vi "Do_Every_minute.vi"(1 "Ch Names":string[](array[string]), 2 "Values":dbl[](array[numeric]) format="%.2f") -> (0 "Scan Comments":string)   [LabVIEW 2017]
uses:
  Anemometry/Anemometry Sub Vis/Controls/In_Range.ctl
  ADAM Client/Sub VIs/ADAM Controls/Update_scan_value.ctl
  ADAM Client/Sub VIs/ADAM Controls/Traverse_Level_State.ctl
  ADAM Client/Sub VIs/ADAM Controls/Valco_valve_ph.ctl
  <vilib>/Analysis/baseanly.llb/Mean (DBL).vi
  Anemometry/Anemometry Sub Vis/Globals/EnFlo_Tunnel_Global.vi
  ADAM_Global.vi
  <vilib>/Analysis/NI_AALBase.lvlib
panel:
  in  "Kp":dbl=50.0 format="%#_13g"
  in  "Deadband Delta T":dbl=0.002 format="%#_13g"
  out "Max Delta T":dbl(graph)
  in  "Manual Control of Lamps":bool
  out "Power":dbl[][](graph)=[[0.00729, 0.18153463174730816, 0.17352738437348433, 1.6752433719500537, 8.231465735195274, 17.570357598383207, 23.099772817121426, 25.58386930448374, 25.31727725753219, 24.28926231541072, 18.717383219374323, 10.355253339797807, 2.7760273383248344, 0.3109897541921306, 0.08276881403435009, 0.06197], [0.04411, 0.1361526368018142, 0.04039202183336771, 1.5611636795339547, 8.176972694107874, 17.32000974741714, 24.257541358764026, 25.949153465972987, 26.01802540761648, 25.060373307424115, 18.284750328365213, 8.689831176707928, 2.642937641487066, 0.43219350072447926, -0.019957690739617468, 0.07351], [0.05478, 0.03446320268089581, 0.2086595806581808, 1.6919212249796047, 6.580368005180591, 14.333585185483123, 21.06810094963999, 23.709254571137723, 24.04768940379576, 21.01660820522005, 13.60443428327954, 6.2766496258038735, 1.7988963349022484, 0.2952877651784204, 0.05436788410934033, 0.1022], [0.04013, 0.06419557464541133, 0.2035068586120256, 1.3118741659450193, 4.7061387064566835, 9.009825946069038, 12.927700276268434, 17.003135081884164, 16.83885730812343, 12.902263313363814, 8.246161922417906, 4.035269404379355, 1.329605659745338, 0.24574055091433544, 0.012829784119986217, 0.08755], [0.04404, 0.022691144295571734, 0.19102098261858932, 0.8525411026079828, 2.2353542219792946, 3.966676465246214, 6.305347763088489, 8.17672908183636, 7.7348668140659, 5.703994479070454, 3.8329088824353237, 1.9256956625267279, 0.6611488869641811, 0.20508248283573002, 0.10119553469307395, 0.08441]]
  out "Temperature":dbl[][](graph)=[[0.00729, 0.18153463174730816, 0.17352738437348433, 1.6752433719500537, 8.231465735195274, 17.570357598383207, 23.099772817121426, 25.58386930448374, 25.31727725753219, 24.28926231541072, 18.717383219374323, 10.355253339797807, 2.7760273383248344, 0.3109897541921306, 0.08276881403435009, 0.06197], [0.04411, 0.1361526368018142, 0.04039202183336771, 1.5611636795339547, 8.176972694107874, 17.32000974741714, 24.257541358764026, 25.949153465972987, 26.01802540761648, 25.060373307424115, 18.284750328365213, 8.689831176707928, 2.642937641487066, 0.43219350072447926, -0.019957690739617468, 0.07351], [0.05478, 0.03446320268089581, 0.2086595806581808, 1.6919212249796047, 6.580368005180591, 14.333585185483123, 21.06810094963999, 23.709254571137723, 24.04768940379576, 21.01660820522005, 13.60443428327954, 6.2766496258038735, 1.7988963349022484, 0.2952877651784204, 0.05436788410934033, 0.1022], [0.04013, 0.06419557464541133, 0.2035068586120256, 1.3118741659450193, 4.7061387064566835, 9.009825946069038, 12.927700276268434, 17.003135081884164, 16.83885730812343, 12.902263313363814, 8.246161922417906, 4.035269404379355, 1.329605659745338, 0.24574055091433544, 0.012829784119986217, 0.08755], [0.04404, 0.022691144295571734, 0.19102098261858932, 0.8525411026079828, 2.2353542219792946, 3.966676465246214, 6.305347763088489, 8.17672908183636, 7.7348668140659, 5.703994479070454, 3.8329088824353237, 1.9256956625267279, 0.6611488869641811, 0.20508248283573002, 0.10119553469307395, 0.08441]]
  in  "Kp Lamps":dbl=50.0 format="%#_13g"
  in  "Averaging time in Seconds":dbl=200.0 format="%#_13g"
  in  "Disable Sending email to estates regarding Chilled water Temp":bool=TRUE
  in  "Max K Factor":dbl=16.0
  # "Control Parameters"
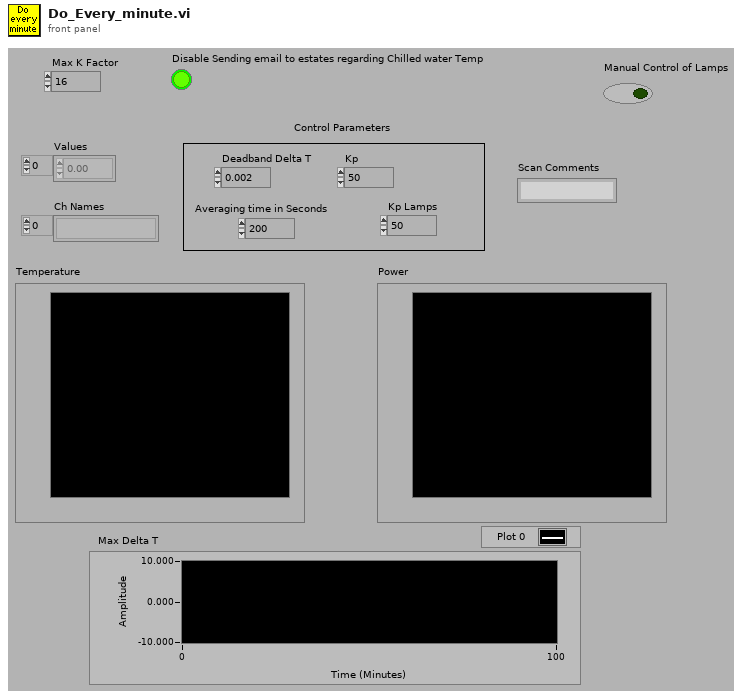
[diagram p1: front panel]
types:
  T1 = typedef "In_Range.ctl" = enum16{"%", "±", "% & ±"}
  T2 = typedef "Update_scan_value.ctl" = cluster{"Channel Name":string, "New Value":dbl}
  T3 = enum16{"Append to Global", "Read Global then Clear"}
  T4 = typedef "Traverse_Level_State.ctl" = enum16{"Running", "Complete"}
  T5 = cluster{"Bus Bar":string, "Connected Items":string[]}
  T6 = cluster{"Ch Name":string, "subarray":string[], "subarray":dbl[], i32, i32}
  T7 = typedef "Client_State_Cluster.ctl" = cluster{"Client Name":string, "Traverse level State":T4, "People to Email":string[], "Next Contact Time":dbl}
  T8 = typedef "Valco_valve_ph.ctl" = u16
  T9 = cluster{"second":i32, "minute":i32, "hour":i32, "day of month":i32, "month":i32, "year":i32, "day of week":i32, "day of year":i32, "is DST":i32}
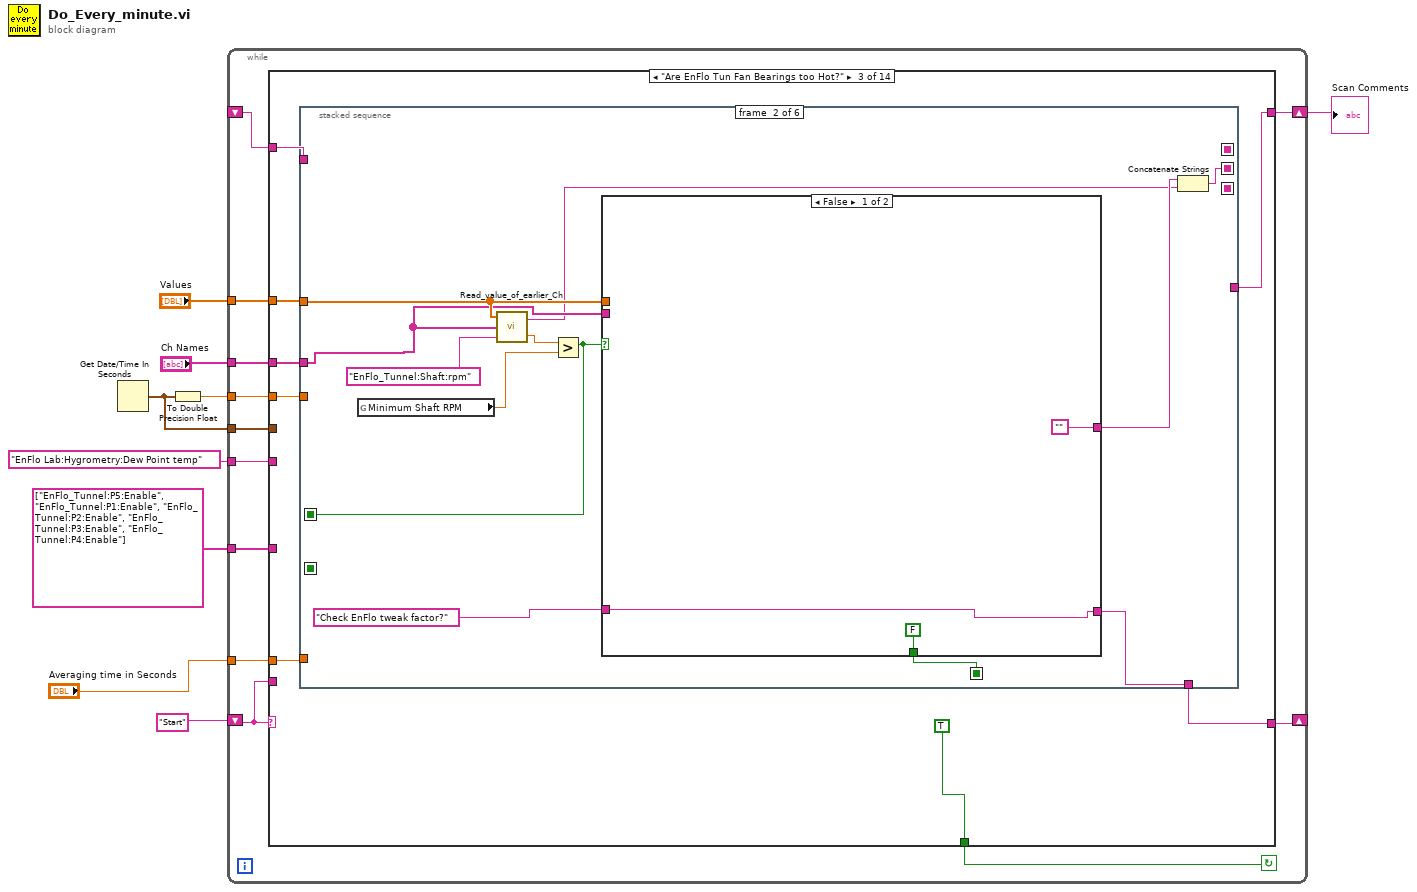
[diagram p0: block diagram]
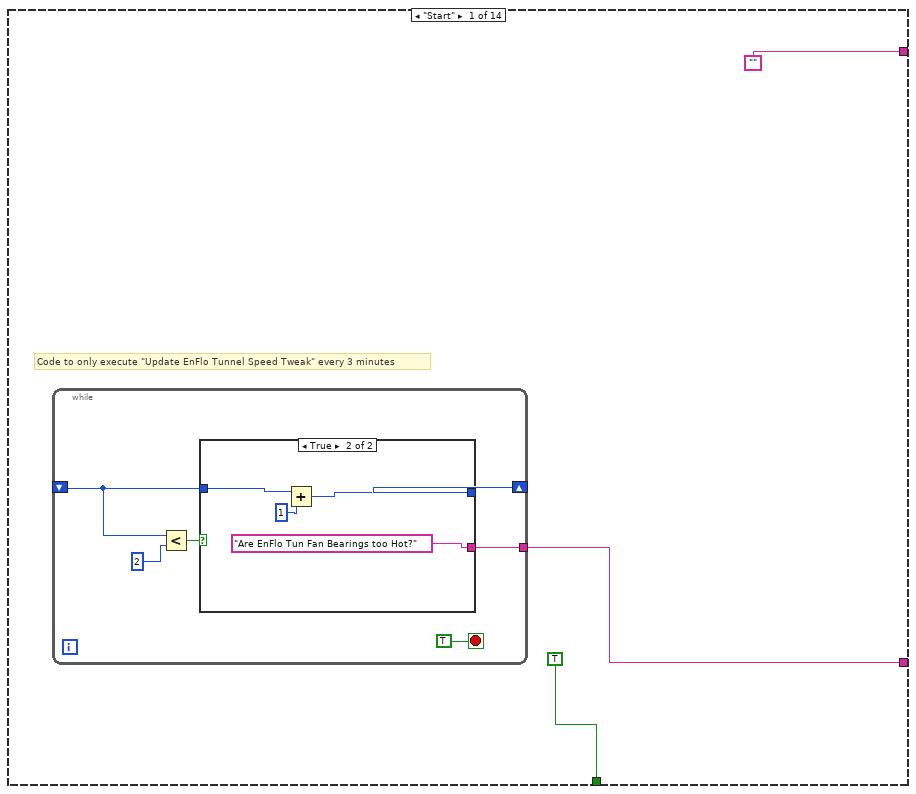
[diagram p2: hidden frame]
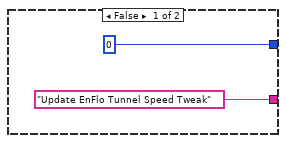
[diagram p3: hidden frame]
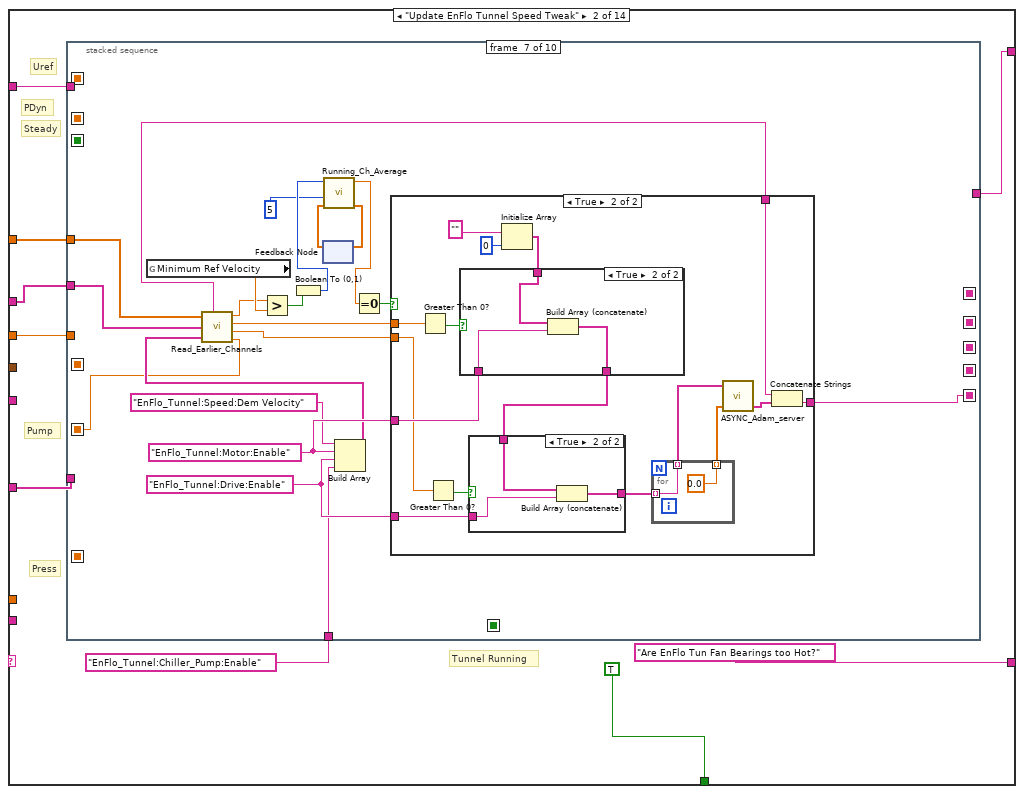
[diagram p4: hidden frame]
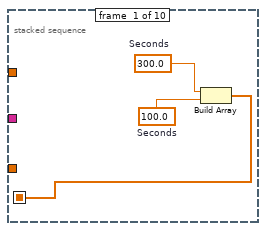
[diagram p5: hidden frame]
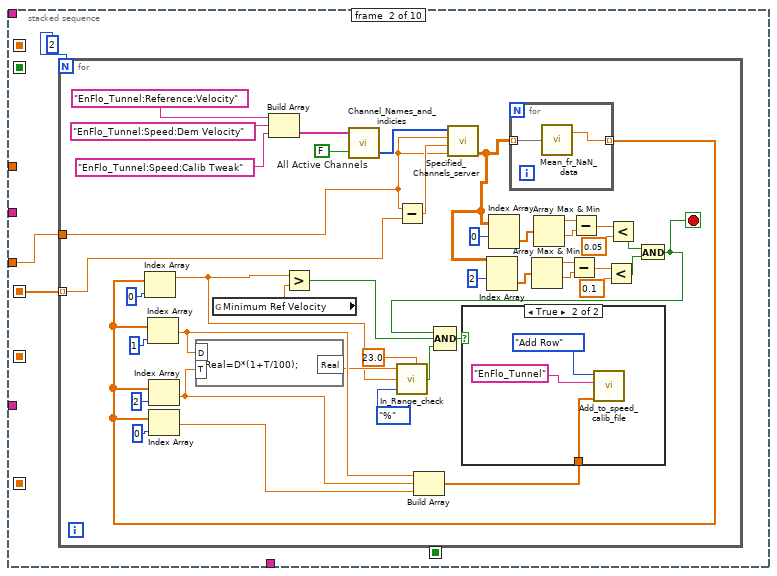
[diagram p6: hidden frame]
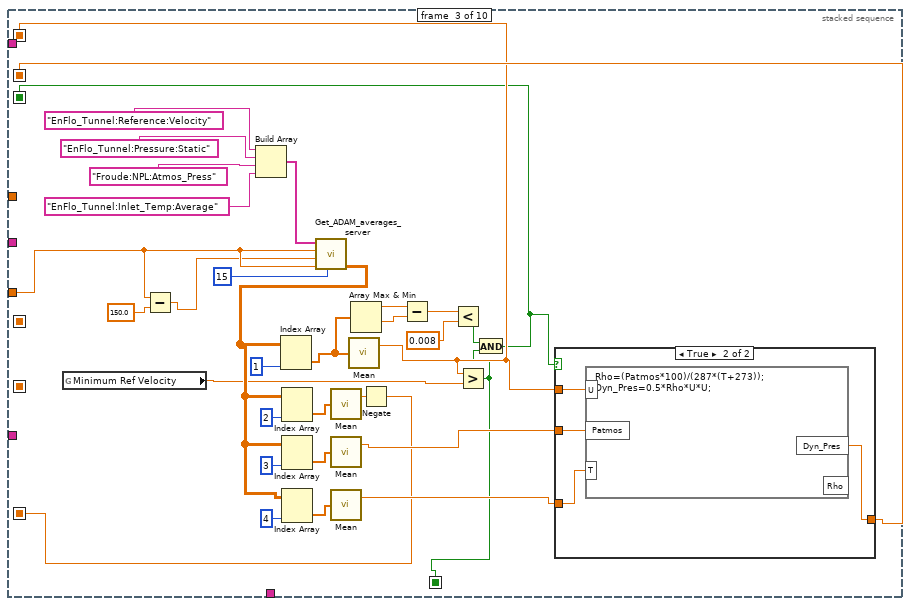
[diagram p8: hidden frame]
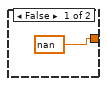
[diagram p9: hidden frame]
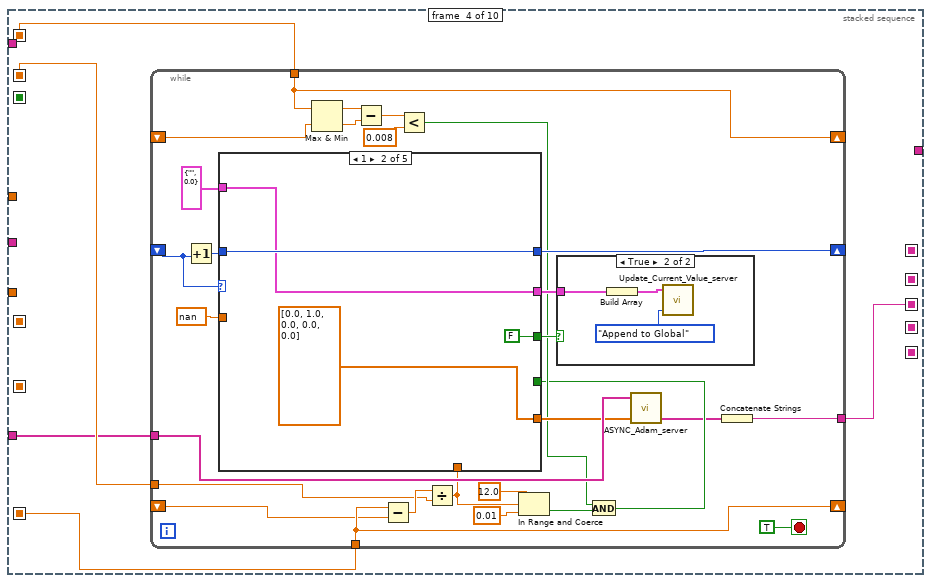
[diagram p10: hidden frame]
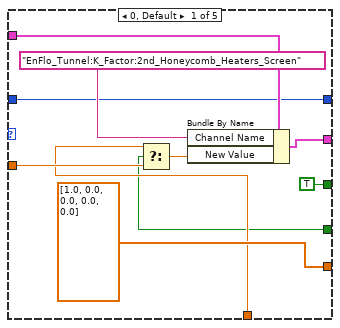
[diagram p12: hidden frame]
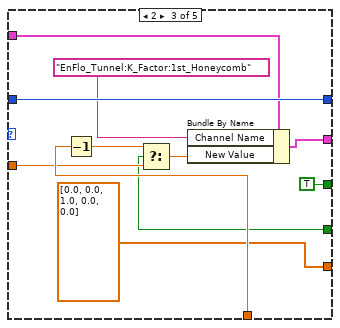
[diagram p13: hidden frame]
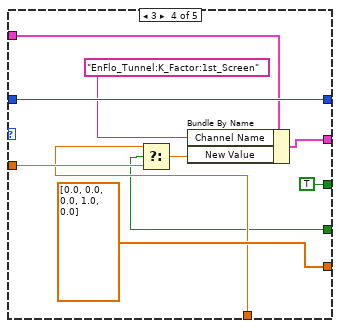
[diagram p14: hidden frame]
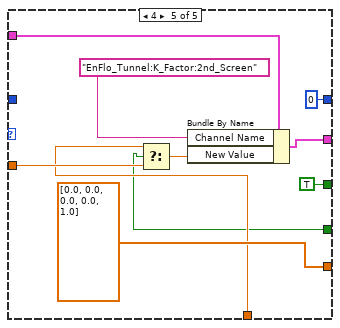
[diagram p15: hidden frame]
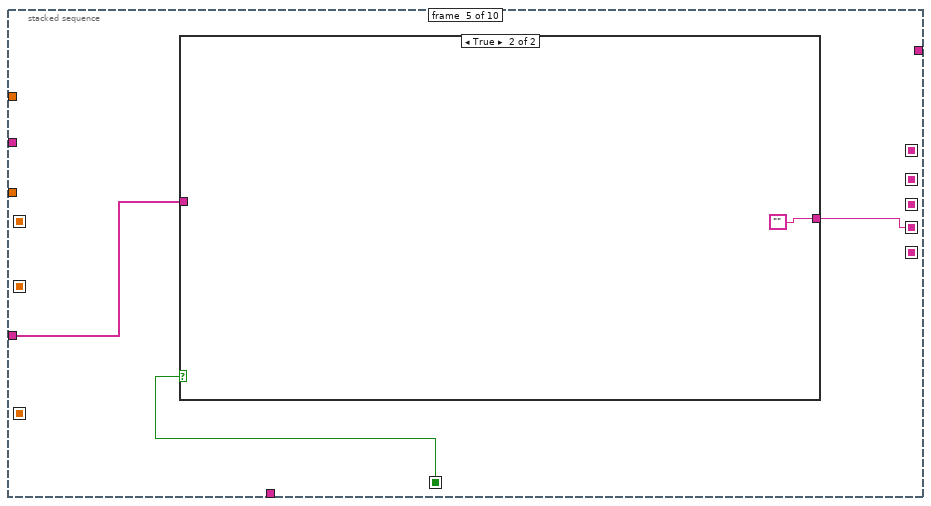
[diagram p16: hidden frame]
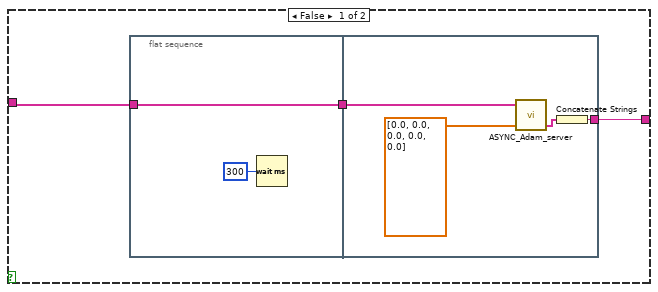
[diagram p17: hidden frame]
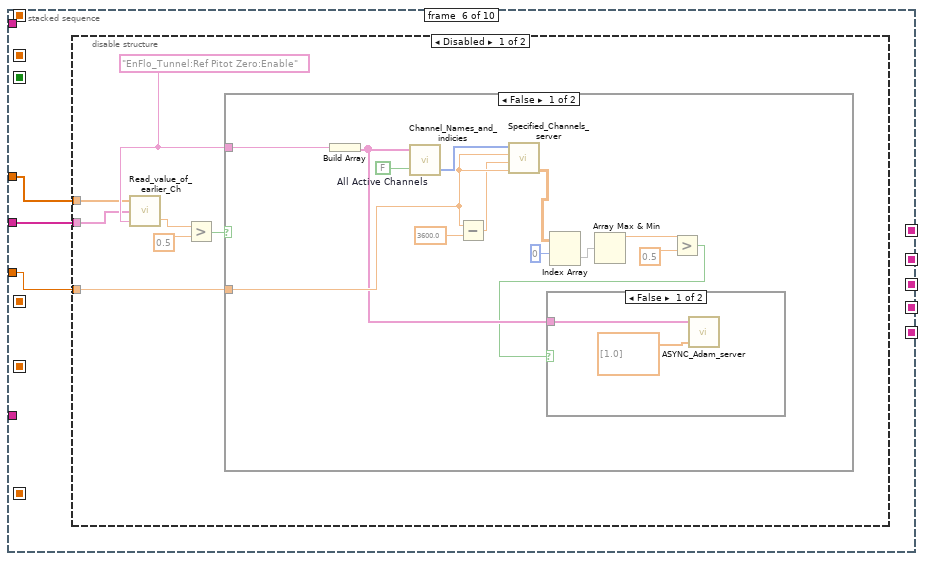
[diagram p18: hidden frame]
diagram:
  n1 = Get Date/Time In Seconds() -> (seconds since 1Jan1904=w5:timestamp)
  n2 = To Double Precision Float(number=w5) -> (double precision float=w6:dbl)
  n3 = while {
    tunnel: "EnFlo Lab:Hygrometry:Dew Point temp" -> [w17]
    tunnel: "Values" -> [w19]
    tunnel: "Ch Names" -> [w20]
    shift-left: "Start" -> [w14]
    shift-right: [w18] -> _
    tunnel: w6 -> [w16]
    tunnel: w5 -> [w15]
    tunnel: string[] ["EnFlo_Tunnel:P5:Enable", "EnFlo_Tunnel:P1:Enable", "EnFlo_Tunnel:P2:Enable", "EnFlo_Tunnel:P3:Enable", "EnFlo_Tunnel:P4:Enable"] -> [w13]
    tunnel: "Averaging time in Seconds" -> [w12]
    shift-right: [w11] -> w1
    shift-left: _ -> [w10]
    stop <- w21 continue-if-true
    n4 = case shown="\"Are EnFlo Tun Fan Bearings too Hot?\"" w14 {
      tunnel: [TRUE TRUE TRUE TRUE TRUE TRUE TRUE TRUE TRUE TRUE TRUE TRUE FALSE FALSE] -> w21
      tunnel: w20 -> [_ w44 w411 w577 _ _ _ w865 w892 w928 w968 w976 w1015 _]
      tunnel: w19 -> [_ w43 w412 w578 _ _ _ w866 w893 w929 w969 w975 w1014 _]
      tunnel: [w23 "Are EnFlo Tun Fan Bearings too Hot?" w410 w576 w805 "Lab Temp Control" "Is Dew point meter Alive?" w869 w880 "More checks" w966 "End" "End" "End"] -> w18
      tunnel: w17 -> [_ _ _ _ _ _ _ w864 _ _ _ _ _ _]
      tunnel: w16 -> [_ w42 w409 w580 _ _ w843 _ _ _ _ w993 w1013 _]
      tunnel: w15 -> [_ _ _ _ _ _ _ _ _ _ _ _ w1016 _]
      tunnel: w14 -> [_ _ _ _ _ _ _ _ _ _ _ _ _ w1094]
      tunnel: w13 -> [_ w40 _ _ _ _ _ _ _ _ _ _ _ _]
      tunnel: w12 -> [_ _ w408 w579 _ _ _ _ _ _ _ _ _ _]
      tunnel: ["" w38 w406 w574 w803 w818 w842 w846 w878 w917 w952 w971 w1007 w1091] -> w11
      tunnel: w10 -> [_ w39 w407 w575 w803 w818 w842 w848 w879 w918 w953 w973 w1008 w1091]
      frame "Start" {
        # "Code to only execute \"Update EnFlo Tunnel Speed Tweak\" every 3 minutes"
        n5 = while {
          shift-right: [w27] -> _
          shift-left: _ -> [w25]
          tunnel: [w26] -> w23
          stop <- TRUE stop-if-true
          n6 = Less?(x=w25, y=2) -> (x < y?=w28:bool)
          n7 = case shown="True" w28 {
            tunnel: [0 w34] -> w27
            tunnel: ["Update EnFlo Tunnel Speed Tweak" "Are EnFlo Tun Fan Bearings too Hot?"] -> w26
            tunnel: w25 -> [_ w35]
            frame False {
            }
            frame True {
              n8 = Add(x=w35, y=1) -> (x+y=w34:i32)
            }
          }
        }
      }
      frame "Update EnFlo Tunnel Speed Tweak" {
        # "Pump"
        # "Tunnel Running"
        # "PDyn"
        # "Steady"
        # "Press"
        # "Uref"
        n9 = stacked-sequence {
          seq-local: [w46 _ _ _ _ _ _ _ _ _] -> [_ w50 _ _ _ _ _ _ _ _]
          seq-local: [_ _ w104 _ _ _ _ _ _ _] -> [_ _ _ w138 _ _ _ _ _ _]
          seq-local: [_ _ w105 _ _ _ _ _ _ _] -> [_ _ _ w140 _ _ _ _ _ _]
          seq-local: [_ _ w102 _ _ _ _ _ _ _] -> [_ _ _ _ _ _ _ _ _ _]
          seq-local: [_ _ w106 _ _ _ _ _ _ _] -> [_ _ _ w139 _ _ _ _ _ _]
          seq-local: [_ _ w101 _ _ _ _ _ _ _] -> [_ _ _ _ w218 _ _ _ w352 _]
          seq-local: [_ _ _ w136 _ _ _ _ _ _] -> [_ _ _ _ _ _ _ _ _ w404]
          seq-local: [_ _ _ _ w217 _ _ _ _ _] -> [_ _ _ _ _ _ _ _ _ w403]
          seq-local: [_ _ _ _ _ _ w258 _ _ _] -> [_ _ _ _ _ _ _ w307 _ _]
          seq-local: [_ _ _ _ _ _ w256 _ _ _] -> [_ _ _ _ _ _ _ _ _ w401]
          seq-local: [_ _ _ _ _ _ _ w303 _ _] -> [_ _ _ _ _ _ _ _ _ w400]
          seq-local: [_ _ _ _ _ _ _ _ w351 _] -> [_ _ _ _ _ _ _ _ _ w399]
          tunnel: w44 -> [_ _ _ _ _ w231 w266 w304 _ _]
          tunnel: w43 -> [_ _ _ _ _ w232 w267 w305 _ _]
          tunnel: w42 -> [_ w49 w130 _ _ w230 _ _ w350 _]
          tunnel: w40 -> [_ _ _ w137 w219 _ _ _ _ _]
          tunnel: w39 -> [_ _ _ _ _ _ _ _ _ w405]
          tunnel: [_ _ _ _ _ _ _ _ _ w402] -> w38
          tunnel: "EnFlo_Tunnel:Chiller_Pump:Enable" ("Desired Ch to Read") -> [_ _ _ _ _ _ w257 _ _ _]
          frame #0 {
            w47 = 100.0  # Seconds
            w48 = 300.0  # Seconds
            n10 = Build Array(w48, w47) -> (w46:dbl[])
          }
          frame #1 {
            n11 = for {
              N: 2 -> [_]
              tunnel: w49 -> [w55]
              tunnel: w50 -> [w54] mode=indexing
              stop <- w53 stop-if-true
              w85 = FALSE  # All Active Channels
              n12 = global read "EnFlo_Tunnel_Global.vi" "Minimum Ref Velocity"() -> (w52:dbl)
              n13 = Build Array("EnFlo_Tunnel:Reference:Velocity", "EnFlo_Tunnel:Speed:Dem Velocity", "EnFlo_Tunnel:Speed:Calib Tweak") -> (w83:string[])
              n14 = call "Channel_Names_and_indicies.vi"("All Active Channels"=w85, "Desired Ch Names"=w83) -> ("Indicies"=w84:i32[])  [unwired: 1 out]
              n15 = Subtract(x=w55, y=w54) -> (x-y=w82:dbl)
              n16 = call "Specified_Channels_server.vi"("End time"=w55, "Start time"=w82, "Clients time"=w55, "Requested channels"=w84) -> ("Output array"=w65:dbl[][])  [unwired: 1 in, 4 out]
              n17 = Index Array(array=w65, index (row)=2 ("Index")) -> (element=w67:dbl[])  [unwired: 1 in]
              n18 = Index Array(array=w65, index (row)=0 ("Index")) -> (element=w80:dbl[])  [unwired: 1 in]
              n19 = for {
                tunnel: w65 -> [w95] mode=indexing
                tunnel: [w94] -> w73 mode=indexing
                n20 = call "Mean_fr_NaN_data.vi"("Data"=w95) -> ("Mean value"=w94:dbl)  [unwired: 1 out]
              }
              n21 = Index Array(array=w73, index=0) -> (element=w59:dbl)
              n22 = Index Array(array=w73, index=1) -> (element=w61:dbl)
              n23 = Index Array(array=w73, index=2) -> (element=w62:dbl)
              n24 = Index Array(array=w73, index=0) -> (element=w72:dbl)
              n25 = formula code="Real=D*(1+T/100);"("D"=w61, "T"=w62) -> ("Real"=w60:dbl)
              n26 = Greater?(x=w59, y=w52) -> (0:w88:bool)
              n27 = call "In_Range_check.vi"("%"=23.0, "Mode"=In_Range."%", "Value"=w59, "Setpoint"=w60) -> ("In Range"=w56:bool)  [unwired: 1 in, 2 out]
              n28 = Build Array(w61, w62, w72) -> (w87:dbl[])
              n29 = Array Max & Min(array=w67) -> (max value=w68:dbl, min value=w69:dbl)  [unwired: 2 out]
              n30 = Array Max & Min(array=w80) -> (max value=w79:dbl, min value=w78:dbl)  [unwired: 2 out]
              n31 = Subtract(x=w68, y=w69) -> (x-y=w70:dbl)
              n32 = Subtract(x=w79, y=w78) -> (x-y=w77:dbl)
              n33 = Less?(x=w70, y=0.1) -> (x < y?=w64:bool)
              n34 = Less?(x=w77, y=0.05) -> (x < y?=w63:bool)
              n35 = And(x=w63, y=w64) -> (x .and. y?=w53:bool)
              n36 = Compound Arithmetic op=AND(w53, w88, w56) -> (w86:bool)
              n37 = case shown="True" w86 {
                tunnel: w87 -> [_ w97]
                frame False {
                }
                frame True {
                  n38 = call "Add_to_speed_calib_file.vi"("New Row"=w97, "Rig Name"="EnFlo_Tunnel" ("y"), "Mode"=enum16{"Add Row", "Get Error Value"}."Add Row") -> ()  [unwired: 3 in, 2 out]
                }
              }
            }
          }
          frame #2 {
            n39 = global read "EnFlo_Tunnel_Global.vi" "Minimum Ref Velocity"() -> (w100:dbl)
            n40 = Subtract(x=w130, y=150.0) -> (x-y=w128:dbl)
            n41 = Build Array("EnFlo_Tunnel:Reference:Velocity", "EnFlo_Tunnel:Pressure:Static", "Froude:NPL:Atmos_Press", "EnFlo_Tunnel:Inlet_Temp:Average") -> (w127:string[])
            n42 = call "Get_ADAM_averages_server.vi"("No of averages"=15, "End time"=w130, "Start time"=w128, "Clients time"=w130, "ADAM Ch Names"=w127) -> ("DBL values"=w109:dbl[][])  [unwired: 1 in, 4 out]
            n43 = Index Array(array=w109, index (col)=1 ("disabled index (col)")) -> (element=w120:dbl[])  [unwired: 1 in]
            n44 = Index Array(array=w109, index (col)=2 ("disabled index (col)")) -> (element=w126:dbl[])  [unwired: 1 in]
            n45 = Index Array(array=w109, index (col)=3 ("disabled index (col)")) -> (element=w112:dbl[])  [unwired: 1 in]
            n46 = Index Array(array=w109, index (col)=4 ("disabled index (col)")) -> (element=w111:dbl[])  [unwired: 1 in]
            n47 = call-poly <vilib>:"Mean.vi"("X"=w126) -> ("mean"=w118:dbl)  [unwired: 1 out]
            n48 = call-poly <vilib>:"Mean.vi"("X"=w112) -> ("mean"=w108:dbl)  [unwired: 1 out]
            n49 = call-poly <vilib>:"Mean.vi"("X"=w111) -> ("mean"=w107:dbl)  [unwired: 1 out]
            n50 = call-poly <vilib>:"Mean.vi"("X"=w120) -> ("mean"=w104:dbl)  [unwired: 1 out]
            n51 = Array Max & Min(array=w120) -> (max value=w121:dbl, min value=w122:dbl)  [unwired: 2 out]
            n52 = Negate(x=w118) -> (-x=w105:dbl)
            n53 = Subtract(x=w121, y=w122) -> (x-y=w123:dbl)
            n54 = Less?(x=w123, y=0.008) -> (x < y?=w103:bool)
            n55 = Greater?(x=w104, y=w100) -> (0:w101:bool)
            n56 = And(x=w103, y=w101) -> (x .and. y?=w102:bool)
            n57 = case shown="True" w102 {
              tunnel: w107 -> [_ w135]
              tunnel: w108 -> [_ w134]
              tunnel: w104 -> [_ w133]
              tunnel: [nan w132] -> w106
              frame False {
              }
              frame True {
                n58 = formula code="Rho=(Patmos*100)/(287*(T+273));\nDyn_Pres=0.5*Rho*U*U;"("Patmos"=w134, "T"=w135, "U"=w133) -> ("Dyn_Pres"=w132:dbl)  [unwired: 1 out]
              }
            }
          }
          frame #3 {
            n59 = while {
              shift-right: [w167] -> _
              shift-left: _ -> [w165]
              shift-right: [w163] -> _
              shift-left: _ -> [w162]
              tunnel: w140 -> [w163]
              tunnel: w139 -> [w160]
              shift-right: [w159] -> _
              shift-left: _ -> [w158]
              tunnel: w138 -> [w159]
              tunnel: w137 -> [w151]
              tunnel: [w141] -> w136
              stop <- TRUE stop-if-true
              n60 = Increment(x=w165) -> (x+1=w166:i32)
              n61 = Max & Min(x=w159, y=w158) -> (max(x,y)=w157:dbl, min(x,y)=w156:dbl)
              n62 = Subtract(x=w157, y=w156) -> (x-y=w155:dbl)
              n63 = Subtract(x=w163, y=w162) -> (x-y=w161:dbl)
              n64 = Less?(x=w155, y=0.008) -> (x < y?=w144:bool)
              n65 = Divide(x=w161, y=w160) -> (x/y=w148:dbl)
              n66 = In Range and Coerce(upper limit=12.0, x=w148, lower limit=0.01) -> (In Range?=w145:bool)  [unwired: 1 out]
              n67 = And(x=w144, y=w145) -> (x .and. y?=w143:bool)
              n68 = case shown="1" w165 {
                tunnel: [w174 w185 w196 w206 0] -> w167
                tunnel: w166 -> [w174 w185 w196 w206 _]
                tunnel: T2 {"Channel Name"="", "New Value"=0.0} ("Update Scan Value Cluster") -> [w181 w184 w195 w205 w216]
                tunnel: w148 -> [w175 _ w193 w199 w210]
                tunnel: [w179 w184 w192 w203 w214] -> w153
                tunnel: nan -> [w178 _ w190 w202 w213]
                tunnel: [dbl[] [1.0, 0.0, 0.0, 0.0, 0.0] ("Values") dbl[] [0.0, 1.0, 0.0, 0.0, 0.0] ("Values") dbl[] [0.0, 0.0, 1.0, 0.0, 0.0] ("Values") dbl[] [0.0, 0.0, 0.0, 1.0, 0.0] ("Values") dbl[] [0.0, 0.0, 0.0, 0.0, 1.0] ("Values")] -> w150
                tunnel: [TRUE FALSE TRUE TRUE TRUE] -> w149
                tunnel: w143 -> [w172 _ w186 w197 w207]
                frame 0, Default {
                  n69 = Select(t=w175, s=w172, f=w178) -> (s? t:f=w177:dbl)
                  n70 = Bundle By Name(cluster=w181, "Channel Name"="EnFlo_Tunnel:K_Factor:2nd_Honeycomb_Heaters_Screen", "New Value"=w177) -> (w179:T2)
                }
                frame 1 {
                }
                frame 2 {
                  n71 = Decrement(x=w193) -> (x-1=w191:dbl)
                  n72 = Select(t=w191, s=w186, f=w190) -> (s? t:f=w189:dbl)
                  n73 = Bundle By Name(cluster=w195, "Channel Name"="EnFlo_Tunnel:K_Factor:1st_Honeycomb", "New Value"=w189) -> (w192:T2)
                }
                frame 3 {
                  n74 = Select(t=w199, s=w197, f=w202) -> (s? t:f=w201:dbl)
                  n75 = Bundle By Name(cluster=w205, "Channel Name"="EnFlo_Tunnel:K_Factor:1st_Screen", "New Value"=w201) -> (w203:T2)
                }
                frame 4 {
                  n76 = Select(t=w210, s=w207, f=w213) -> (s? t:f=w212:dbl)
                  n77 = Bundle By Name(cluster=w216, "Channel Name"="EnFlo_Tunnel:K_Factor:2nd_Screen", "New Value"=w212) -> (w214:T2)
                }
              }
              n78 = case shown="True" w149 {
                tunnel: w153 -> [_ w169]
                frame False {
                }
                frame True {
                  n79 = Build Array(w169) -> (w170:T2[])
                  n80 = call "Update_Current_Value_server.vi"("Mode"=T3."Append to Global", "Update array in"=w170) -> ()  [unwired: 1 in, 1 out]
                }
              }
              n81 = call "ASYNC_Adam_server.vi"("Values"=w150, "Channel Names"=w151) -> ("Scan Comments"=w142:string[])  [unwired: 1 in, 2 out]
              n82 = Concatenate Strings(w142) -> (w141:string)
            }
          }
          frame #4 {
            n83 = case shown="True" w218 {
              tunnel: w219 -> [w222 _]
              tunnel: [w220 ""] -> w217
              frame False {
                n84 = flat-sequence {
                  tunnel: w222 -> [w224]
                  tunnel: [w224] -> w221
                  tunnel: w221 -> [w227]
                  tunnel: [w225] -> w220
                  frame #0 {
                    n85 = Wait (ms)(milliseconds to wait=u32 300) -> ()  [unwired: 1 out]
                  }
                  frame #1 {
                    n86 = call "ASYNC_Adam_server.vi"("Values"=dbl[] [0.0, 0.0, 0.0, 0.0, 0.0], "Channel Names"=w227) -> ("Scan Comments"=w226:string[])  [unwired: 1 in, 2 out]
                    n87 = Concatenate Strings(w226) -> (w225:string)
                  }
                }
              }
              frame True {
              }
            }
          }
          frame #5 {
            n88 = disable-structure shown="Disabled" {
              disable-tunnel: w232 -> [w235 _]
              disable-tunnel: w231 -> [w234 _]
              disable-tunnel: w230 -> [w233 _]
              frame Disabled {
                w236 = "EnFlo_Tunnel:Ref Pitot Zero:Enable"
                n89 = call "Read_value_of_earlier_Ch.vi"("Desired Ch to Read"=w236, "Ch names"=w234, "Present scan array"=w235) -> ("Value"=w238:dbl)  [unwired: 1 in, 1 out]
                n90 = Greater?(x=w238, y=0.5) -> (0:w239:bool)
                n91 = case shown="False" w239 {
                  tunnel: w233 -> [w252 _]
                  tunnel: w236 -> [w242 _]
                  frame False {
                    w251 = FALSE  # All Active Channels
                    n92 = Build Array(w242) -> (w241:string[])
                    n93 = call "Channel_Names_and_indicies.vi"("All Active Channels"=w251, "Desired Ch Names"=w241) -> ("Indicies"=w250:i32[])  [unwired: 1 out]
                    n94 = Subtract(x=w252, y=3600.0) -> (x-y=w249:dbl)
                    n95 = call "Specified_Channels_server.vi"("End time"=w252, "Start time"=w249, "Clients time"=w252, "Requested channels"=w250) -> ("Output array"=w246:dbl[][])  [unwired: 1 in, 4 out]
                    n96 = Index Array(array=w246, index (row)=0 ("Index")) -> (element=w247:dbl[])  [unwired: 1 in]
                    n97 = Array Max & Min(array=w247) -> (max value=w244:dbl)  [unwired: 3 out]
                    n98 = Greater?(x=w244, y=0.5) -> (0:w240:bool)
                    n99 = case shown="False" w240 {
                      tunnel: w241 -> [w253 _]
                      frame False {
                        n100 = call "ASYNC_Adam_server.vi"("Values"=dbl[] [1.0], "Channel Names"=w253) -> ()  [unwired: 1 in, 3 out]
                      }
                      frame True {
                      }
                    }
                  }
                  frame True {
                  }
                }
              }
              frame Enabled {
              }
            }
          }
          frame #6 {
            w273 = "EnFlo_Tunnel:Drive:Enable" ("Desired Ch to Read")
            w271 = "EnFlo_Tunnel:Motor:Enable" ("Desired Ch to Read")
            n101 = global read "EnFlo_Tunnel_Global.vi" "Minimum Ref Velocity"() -> (w275:dbl)
            n102 = feedback #1() -> (w263:dbl[])  [unwired: 1 in]
            n103 = Build Array("EnFlo_Tunnel:Speed:Dem Velocity" ("Desired Ch to Read"), w271, w273, w257) -> (w269:string[])
            n104 = call "Read_Earlier_Channels.vi"("Present scan array"=w267, "Ch names"=w266, "Desired Channels"=w269) -> ("Scan comments"=w255:string, "Index 0"=w274:dbl, "Index 1"=w270:dbl, "Index 2"=w272:dbl, "Index 3"=w258:dbl)  [unwired: 1 out]
            n105 = Greater?(x=w274, y=w275) -> (0:w265:bool)
            n106 = Boolean To (0,1)(Boolean=w265) -> (0, 1=w262:i16)
            n107 = call "Running_Ch_Average.vi"("Shift In"=w263, "History length"=5, "New Value"=w262) -> ("Shift Out"=w264:dbl[], "mean"=w259:dbl)  [unwired: 3 in]
            n108 = feedback-in #1(w264) -> ()
            n109 = Equal To 0?(x=w259) -> (x = 0?=w260:bool)
            n110 = case shown="True" w260 {
              tunnel: w270 -> [_ w292]
              tunnel: w271 -> [_ w287]
              tunnel: w272 -> [_ w286]
              tunnel: w273 -> [_ w283]
              tunnel: [w276 w278] -> w256
              tunnel: w255 -> [w276 w277]
              frame False {
              }
              frame True {
                n111 = Greater Than 0?(x=w292) -> (x > 0?=w291:bool)
                n112 = Greater Than 0?(x=w286) -> (x > 0?=w285:bool)
                n113 = Initialize Array("", 0 ("dimension size")) -> (w288:string[])
                n114 = case shown="True" w291 {
                  tunnel: w288 -> [w299 w302]
                  tunnel: w287 -> [_ w301]
                  tunnel: [w299 w300] -> w284
                  frame False {
                  }
                  frame True {
                    n115 = Build Array (concatenate)(w302, w301) -> (w300:string[])
                  }
                }
                n116 = case shown="True" w285 {
                  tunnel: w284 -> [w295 w298]
                  tunnel: w283 -> [_ w297]
                  tunnel: [w295 w296] -> w281
                  frame False {
                  }
                  frame True {
                    n117 = Build Array (concatenate)(w298, w297) -> (w296:string[])
                  }
                }
                n118 = for {
                  tunnel: [w294] -> w282 mode=indexing
                  tunnel: w281 -> [w294] mode=indexing
                  tunnel: [0.0] -> w280 mode=indexing
                }
                n119 = call "ASYNC_Adam_server.vi"("Values"=w280, "Channel Names"=w282) -> ("Scan Comments"=w279:string[])  [unwired: 1 in, 2 out]
                n120 = Concatenate Strings(w277, w279) -> (w278:string)
              }
            }
          }
          frame #7 {
            n121 = Greater?(x=w307, y=0.5) -> (0:w306:bool)
            n122 = case shown="True" w306 {
              tunnel: w305 -> [_ w329]
              tunnel: w304 -> [_ w328]
              tunnel: ["" w310] -> w303
              frame False {
              }
              frame True {
                w315 = errorcluster {"status"=FALSE, "code"=0, "source"=""} ("error in (no error)")
                w319 = TRUE ("In Range")
                w314 = string[] ["EnFlo_Tunnel:Power:Chiller_Pump_Exchanger", "EnFlo_Tunnel:Meas Power:Chiller_Pump_Exchanger", "EnFlo_Tunnel:Power:Chiller_Pump_Floor", "EnFlo_Tunnel:Meas Power:Chiller_Pump_Floor"]
                n123 = call "Read_Earlier_Channels.vi"("Present scan array"=w329, "Ch names"=w328, "Desired Channels"=w314) -> ("Scan comments"=w310:string, "Index 0"=w317:dbl, "Index 1"=w316:dbl, "Index 2"=w313:dbl, "Index 3"=w312:dbl)  [unwired: 1 out]
                n124 = call "In_Range_check.vi"("±"=6.0, "Mode"=In_Range."±", "Value"=w312, "Setpoint"=w313) -> ("In Range"=w321:bool)  [unwired: 3 in]
                n125 = call "In_Range_check.vi"("±"=6.0, "Mode"=In_Range."±", "Value"=w316, "Setpoint"=w317) -> ("In Range"=w323:bool)  [unwired: 3 in]
                n126 = feedback-in #2(w323) -> ()
                n127 = feedback #2(w319) -> (w322:bool)
                n128 = feedback #3(w319) -> (w320:bool)
                n129 = feedback-in #3(w321) -> ()
                n130 = Or(x=w321, y=w320) -> (x .or. y?=w311:bool)
                n131 = Or(x=w323, y=w322) -> (x .or. y?=w318:bool)
                n132 = case shown="False" w318 {
                  tunnel: w315 -> [_ _]
                  tunnel: w314 -> [w349 _]
                  tunnel: w317 -> [w346 _]
                  tunnel: w316 -> [w345 _]
                  frame False {
                    n133 = Index Array(array=w349, index #1=0 ("index"), index #2=1 ("index")) -> (element #1=w341:string, element #2=w343:string)
                    n134 = Format Into String(format string="Warning\n%s=%d %s=%d", w341, w346, w343, w345) -> (resulting string=w340:string)  [unwired: 2 in, 1 out]
                    n135 = call "Server_Emails.vi"("Client Name Contains"="EnFlo_Tunnel", "Message"=w340, "Subject"=w341) -> ()  [unwired: 2 in, 3 out]
                  }
                  frame True {
                  }
                }
                n136 = case shown="False" w311 {
                  tunnel: w315 -> [_ _]
                  tunnel: w314 -> [w339 _]
                  tunnel: w313 -> [w336 _]
                  tunnel: w312 -> [w335 _]
                  frame False {
                    n137 = Index Array(array=w339, index #1=0 ("index"), index #2=1 ("index")) -> (element #1=w331:string, element #2=w333:string)
                    n138 = Format Into String(format string="Warning\n%s=%d %s=%d", w331, w336, w333, w335) -> (resulting string=w330:string)  [unwired: 2 in, 1 out]
                    n139 = call "Server_Emails.vi"("Client Name Contains"="EnFlo_Tunnel", "Message"=w330, "Subject"=w331) -> ()  [unwired: 2 in, 3 out]
                  }
                  frame True {
                  }
                }
              }
            }
          }
          frame #8 {
            n140 = case shown="True" w352 {
              tunnel: w350 -> [_ w357]
              tunnel: ["" w358] -> w351
              tunnel: w350 -> [_ w355]
              tunnel: w350 -> [_ w354]
              frame False {
              }
              frame True {
                w359 = string[] ["EnFlo_Tunnel:Temp:Pre_Inlet_Y=1500_Z=450", "EnFlo_Tunnel:Temp:Pre_Inlet_Y=-1500_Z=450", "EnFlo_Tunnel:Temp:Pre_Inlet_Y=1000_Z=450", "EnFlo_Tunnel:Temp:Pre_Inlet_Y=-1000_Z=450", "EnFlo_Tunnel:Temp:Pre_Inlet_Y=500_Z=450"] ("Sub set")
                n141 = Subtract(x=w357, y=300.0 ("x-y")) -> (x-y=w371:dbl)
                n142 = call "Get_ADAM_averages_client.vi"("No of averages"=1, "End time"=w357, "Start time"=w371, "ADAM Ch Names"=w359) -> ("Messages"=w358:string, "DBL values"=w375:dbl[][])  [unwired: 3 in, 3 out]
                n143 = Index Array(array=w375, index (row)=1 ("disabled index (col)")) -> (element=w370:dbl[])  [unwired: 1 in]
                n144 = Array Subset(array=w370, index=1, length=5) -> (w368:dbl[])
                n145 = Array Max & Min(array=w368) -> (max value=w365:dbl, max index (indices)=w363:i32, min value=w367:dbl, min index (indices)=w364:i32)
                n146 = Subtract(x=w365, y=w367) -> (x-y=w360:dbl)
                n147 = Index Array(array=w359, index=w364) -> (element=w361:string)
                n148 = Greater Or Equal?(x=w360, y=0.3) -> (x >= y?=w356:bool)
                n149 = Index Array(array=w359, index=w363) -> (element=w362:string)
                n150 = case shown="True" w356 {
                  tunnel: w362 -> [_ w391]
                  tunnel: w361 -> [_ w390]
                  tunnel: w360 -> [_ w389]
                  tunnel: w355 -> [_ w381]
                  tunnel: w354 -> [_ w379]
                  frame False {
                  }
                  frame True {
                    n151 = Subtract(x=w381, y=1200.0) -> (x-y=w384:dbl)
                    n152 = call "Get_ADAM_averages_client.vi"("No of averages"=20, "End time"=w379, "Start time"=w384, "ADAM Ch Names"=string[] ["EnFlo_Tunnel:Reference:Velocity"]) -> ("DBL values"=w387:dbl[][])  [unwired: 3 in, 4 out]
                    n153 = global read "EnFlo_Tunnel_Global.vi" "Minimum Ref Velocity for taking Results"() -> (w385:dbl)
                    n154 = Index Array(array=w387, index (col)=1 ("disabled index (col)")) -> (element=w386:dbl[])  [unwired: 1 in]
                    n155 = Greater Or Equal?(x=w386, y=w385) -> (x >= y?=w388:bool[])
                    n156 = And Array Elements(Boolean array=w388) -> (logical AND=w377:bool)
                    n157 = case shown="True" w377 {
                      tunnel: w389 -> [_ w394]
                      tunnel: w390 -> [_ w393]
                      tunnel: w391 -> [_ w392]
                      frame False {
                      }
                      frame True {
                        n158 = Format Into String(format string="The %s is %.2f degC more than %s.\\n Check the inlet fans are operating correctly." ("Format String"), w392, w394, w393) -> (resulting string=w396:string)  [unwired: 2 in, 1 out]
                        n159 = call "Server_Emails.vi"("Client Name Contains"="EnFlo_Tunnel", "Message"=w396, "Subject"="Large Inlet Temperature Variation" ("Error Type")) -> ()  [unwired: 2 in, 3 out]
                      }
                    }
                  }
                }
              }
            }
          }
          frame #9 {
            n160 = Concatenate Strings(w405, w403, w404, w401, w400, w399) -> (w402:string)
          }
        }
      }
      frame "Are EnFlo Tun Fan Bearings too Hot?" {
        n161 = stacked-sequence {
          seq-local: [_ w455 _ _ _ _] -> [_ _ w486 _ _ _]
          seq-local: [w414 _ _ _ _ _] -> [_ _ _ _ _ w572]
          seq-local: [_ _ w485 _ _ _] -> [_ _ _ _ _ w570]
          seq-local: [_ w451 _ _ _ _] -> [_ _ _ _ _ w571]
          seq-local: [_ w450 _ _ _ _] -> [_ _ _ w506 _ _]
          seq-local: [_ _ _ w505 _ _] -> [_ _ _ _ w520 _]
          tunnel: w412 -> [w424 w458 w488 w508 w519 _]
          tunnel: w411 -> [w423 w457 w487 w507 w518 _]
          tunnel: [_ w459 _ _ _ _] -> w410
          tunnel: w409 -> [_ _ _ _ w517 _]
          tunnel: w408 -> [_ _ _ _ w516 _]
          tunnel: w407 -> [_ _ _ _ _ w573]
          tunnel: [_ _ _ _ _ w569] -> w406
          frame #0 {
            n162 = Build Array("EnFlo_Tunnel:Reference:Velocity", "EnFlo_Tunnel:Fan Gearbox:Y+ Temp", "EnFlo_Tunnel:Fan Gearbox:Y- Temp") -> (w422:string[])
            n163 = while {
              tunnel: [w429] -> w415
              tunnel: [w430] -> w416
              tunnel: [w438] -> w421
              shift-left: _ -> [w438]
              shift-right: [w431] -> w420
              tunnel: w422 -> [w441]
              tunnel: w423 -> [w442]
              tunnel: w424 -> [w443]
              tunnel: [w427] -> _
              tunnel: [w426] -> w414
              stop <- FALSE continue-if-true
              n164 = call "Read_Earlier_Channels.vi"("Present scan array"=w443, "Ch names"=w442, "Desired Channels"=w441) -> ("Scan comments"=w426:string, "Index 0"=w427:dbl, "Index 1"=w430:dbl, "Index 2"=w429:dbl)  [unwired: 2 out]
              n165 = Select(t=60.0, s=w438, f=63.0) -> (s? t:f=w437:dbl)
              n166 = Greater?(x=w430, y=w437) -> (0:w435:bool)
              n167 = Greater?(x=w429, y=w437) -> (0:w434:bool)
              n168 = Less?(x=w427, y=2.55) -> (x < y?=w433:bool)
              n169 = Compound Arithmetic op=OR(w435, w434) -> (w432:bool)
              n170 = Compound Arithmetic op=AND(w433, w432) -> (w431:bool)
            }
            n171 = Compound Arithmetic op=AND(invert w421, w420) -> (w419:bool)
            n172 = case shown="True" w419 {
              tunnel: w416 -> [_ w447]
              tunnel: w415 -> [_ w444]
              frame False {
              }
              frame True {
                n173 = Format Into String(format string="The fan gearbox temperatures on the EnFlo Tunnel are %.1f and %.1f deg C instead of about 58 deg C. They may well be running low on oil, if so, there will probably be a squealing sound coming from the fan unit. You should stop the tunnel as soon as possible to prevent the bearings becoming wrecked." ("Format String"), w447, w444) -> (resulting string=w446:string)  [unwired: 2 in, 1 out]
                n174 = call "Server_Emails.vi"("Client Name Contains"="EnFlo_Tunnel", "Message"=w446, "Subject"="Bearings Too Hot" ("Error Type")) -> ()  [unwired: 2 in, 3 out]
              }
            }
          }
          frame #1 {
            n175 = global read "EnFlo_Tunnel_Global.vi" "Minimum Shaft RPM"() -> (w454:dbl)
            n176 = call "Read_value_of_earlier_Ch.vi"("Desired Ch to Read"="EnFlo_Tunnel:Shaft:rpm", "Ch names"=w457, "Present scan array"=w458) -> ("Value"=w461:dbl, "Scan comment"=w452:string)  [unwired: 1 in]
            n177 = Greater?(x=w461, y=w454) -> (0:w450:bool)
            n178 = case shown="False" w450 {
              tunnel: [w464 w477] -> w459
              tunnel: w458 -> [_ w475]
              tunnel: w457 -> [_ w474]
              tunnel: "Check EnFlo tweak factor?" -> [w464 w476]
              tunnel: [FALSE w468] -> w455
              tunnel: ["" w465] -> w453
              frame False {
              }
              frame True {
                n179 = call "Read_value_of_earlier_Ch.vi"("Desired Ch to Read"="EnFlo_Tunnel:Heater:Enable", "Ch names"=w474, "Present scan array"=w475) -> ("Value"=w472:dbl, "Scan comment"=w467:string)  [unwired: 1 in]
                n180 = call "Read_value_of_earlier_Ch.vi"("Desired Ch to Read"="EnFlo_Tunnel:Enable:Inlet_Lamps", "Ch names"=w474, "Present scan array"=w475) -> ("Value"=w471:dbl, "Scan comment"=w466:string)  [unwired: 1 in]
                n181 = Build Array(w472, w471) -> (w470:dbl[])
                n182 = Greater?(x=w470, y=0.5) -> (0:w469:bool[])
                n183 = And Array Elements(Boolean array=w469) -> (logical AND=w468:bool)
                n184 = case shown="True" w468 {
                  tunnel: [w480 w481] -> w477
                  tunnel: w476 -> [w480 w484]
                  frame False {
                  }
                  frame True {
                    n185 = Select(t=w484, s="Manual Control of Lamps", f="Lamp control") -> (s? t:f=w481:string)
                  }
                }
                n186 = Concatenate Strings(w467, w466) -> (w465:string)
              }
            }
            n187 = Concatenate Strings(w453, w452) -> (w451:string)
          }
          frame #2 {
            n188 = case shown="False" w486 {
              tunnel: w488 -> [w493 _]
              tunnel: w487 -> [w492 _]
              tunnel: [w489 ""] -> w485
              frame False {
                n189 = for {
                  tunnel: [w499] -> w496 mode=indexing if=w500
                  tunnel: [0.0 ("Value")] -> w495 mode=indexing if=w500
                  tunnel: string[] ["EnFlo_Tunnel:Inlet_Lamp Y=-1313_Z=1125:Dem_Power(%)", "EnFlo_Tunnel:Inlet_Lamp Y=-1313_Z=375:Dem_Power(%)", "EnFlo_Tunnel:Inlet_Lamp Y=-438_Z=1125:Dem_Power(%)", "EnFlo_Tunnel:Inlet_Lamp Y=-438_Z=375:Dem_Power(%)", "EnFlo_Tunnel:Inlet_Lamp Y=438_Z=1125:Dem_Power(%)", "EnFlo_Tunnel:Inlet_Lamp Y=438_Z=375:Dem_Power(%)", "EnFlo_Tunnel:Inlet_Lamp Y=1313_Z=1125:Dem_Power(%)", "EnFlo_Tunnel:Inlet_Lamp Y=1313_Z=375:Dem_Power(%)"] ("Sub set") -> [w499] mode=indexing
                  tunnel: w493 -> [w503]
                  tunnel: w492 -> [w502]
                  tunnel: [w497] -> w491 mode=indexing
                  n190 = call "Read_value_of_earlier_Ch.vi"("Desired Ch to Read"=w499, "Ch names"=w502, "Present scan array"=w503) -> ("Value"=w501:dbl, "Scan comment"=w497:string)  [unwired: 1 in]
                  n191 = Not Equal To 0?(x=w501) -> (x != 0?=w500:bool)
                }
                n192 = call "ASYNC_Adam_server.vi"("Values"=w495, "Channel Names"=w496) -> ("Scan Comments"=w490:string[])  [unwired: 1 in, 2 out]
                n193 = Concatenate Strings(w491, w490) -> (w489:string)
              }
              frame True {
              }
            }
          }
          frame #3 {
            n194 = case shown="True" w506 {
              tunnel: w508 -> [_ w513]
              tunnel: w507 -> [_ w512]
              tunnel: [FALSE w510] -> w505
              frame False {
              }
              frame True {
                n195 = call "Read_value_of_earlier_Ch.vi"("Desired Ch to Read"="EnFlo_Tunnel:Heater:Enable", "Ch names"=w512, "Present scan array"=w513) -> ("Value"=w515:dbl)  [unwired: 1 in, 1 out]
                n196 = Greater?(x=w515, y=0.5) -> (0:w510:bool)
              }
            }
          }
          frame #4 {
            n197 = case shown="True" w520 {
              tunnel: w517 -> [_ w524]
              tunnel: w519 -> [_ w523]
              tunnel: w518 -> [_ w522]
              tunnel: w516 -> [_ w521]
              frame False {
              }
              frame True {
                n198 = stacked-sequence {
                  seq-local: [w529 _] -> [_ w546]
                  seq-local: [w528 _] -> [_ w549]
                  tunnel: w524 -> [w544 _]
                  tunnel: w523 -> [_ w548]
                  tunnel: w522 -> [_ w547]
                  tunnel: w521 -> [w525 _]
                  frame #0 {
                    w532 = 2.0 ("y")
                    # "Delta T"
                    n199 = Subtract(x=w544, y=w525) -> (x-y=w543:dbl)
                    n200 = call "Get_ADAM_averages_server.vi"("No of averages"=1, "End time"=w544, "Start time"=w543, "Clients time"=w544, "ADAM Ch Names"=string[] ["EnFlo_Tunnel:Temp:Pre_Inlet_Y=-1500_Z=450", "EnFlo_Tunnel:Temp:Pre_Inlet_Y=-1000_Z=450", "EnFlo_Tunnel:Temp:Pre_Inlet_Y=1500_Z=450", "EnFlo_Tunnel:Temp:Pre_Inlet_Y=1000_Z=450"]) -> ("DBL values"=w541:dbl[][])  [unwired: 1 in, 4 out]
                    n201 = Index Array(array=w541, index (row)=0) -> (element=w539:dbl[])  [unwired: 1 in]
                    n202 = Index Array(array=w539) -> (element #2=w537:dbl, element #3=w538:dbl, element #4=w536:dbl, element #5=w535:dbl)  [unwired: 5 in, 1 out]
                    n203 = Add(x=w537, y=w538) -> (x+y=w534:dbl)
                    n204 = Add(x=w536, y=w535) -> (x+y=w533:dbl)
                    n205 = Divide(x=w534, y=w532) -> (x/y=w526:dbl)
                    n206 = Divide(x=w533, y=w532) -> (x/y=w527:dbl)
                    n207 = Subtract(x=w526, y=w527) -> (x-y=w529:dbl)
                    n208 = Absolute Value(x=w529) -> (abs(x)=w531:dbl)
                    n209 = Greater?(x=w531, y="Deadband Delta T") -> (0:w528:bool)
                  }
                  frame #1 {
                    n210 = case shown="True" w549 {
                      tunnel: w548 -> [_ w568]
                      tunnel: w547 -> [_ w567]
                      tunnel: w546 -> [_ w566]
                      frame False {
                      }
                      frame True {
                        w556 = "EnFlo_Tunnel:Power:Inlet_Door_Heaters" ("Desired Ch to Read")
                        n211 = Multiply(x=w566, y="Kp") -> (x*y=w564:dbl)
                        n212 = In Range and Coerce(upper limit=1.0, x=w564, lower limit=-1.0) -> (coerced(x)=w560:dbl)  [unwired: 1 out]
                        n213 = call "Read_value_of_earlier_Ch.vi"("Desired Ch to Read"=w556, "Ch names"=w567, "Present scan array"=w568) -> ("Value"=w561:dbl)  [unwired: 1 in, 1 out]
                        n214 = Add(x=w561, y=w560) -> (x+y=w557:dbl)
                        n215 = In Range and Coerce(upper limit=90.0, x=w557, lower limit=0.0) -> (coerced(x)=w552:dbl)  [unwired: 1 out]
                        n216 = Not A Number/Path/Refnum?(number/path/refnum=w552) -> (NaN/Path/Refnum?=w553:bool)
                        n217 = Select(t=0.0, s=w553, f=w552) -> (s? t:f=w550:dbl)
                        n218 = Build Array(w556) -> (w555:string[])
                        n219 = Build Array(w550) -> (w554:dbl[])
                        n220 = call "ASYNC_Adam_server.vi"("Values"=w554, "Channel Names"=w555) -> ()  [unwired: 1 in, 3 out]
                      }
                    }
                  }
                }
              }
            }
          }
          frame #5 {
            n221 = Concatenate Strings(w573, w572, w571, w570) -> (w569:string)
          }
        }
      }
      frame "Lamp control" {
        # "Heaters\nOn"
        # "Inlet"
        n222 = stacked-sequence {
          seq-local: [_ _ w611 _ _ _ _] -> [_ _ _ _ _ w700 w774]
          seq-local: [_ _ w609 _ _ _ _] -> [_ _ _ w663 w673 w699 _]
          seq-local: [_ _ _ w660 _ _ _] -> [_ _ _ _ w671 w698 _]
          seq-local: [_ _ _ _ _ w691 _] -> [_ _ _ _ _ _ w763]
          seq-local: [_ w602 _ _ _ _ _] -> [_ _ _ _ _ w697 w757]
          seq-local: [w584 _ _ _ _ _ _] -> [_ _ _ _ w674 w686 _]
          seq-local: [w583 _ _ _ _ _ _] -> [_ _ w607 _ w672 _ _]
          seq-local: [_ _ _ _ w670 _ _] -> [_ _ _ _ _ w685 _]
          seq-local: [w582 _ _ _ _ _ _] -> [_ _ _ _ _ _ w745]
          tunnel: w580 -> [_ _ _ w665 _ _ _]
          tunnel: w579 -> [_ _ _ w664 _ _ _]
          tunnel: w578 -> [w588 _ _ _ _ _ w773]
          tunnel: w577 -> [w587 _ _ _ _ _ w772]
          tunnel: [_ _ _ _ _ _ "Check EnFlo tweak factor?"] -> w576
          tunnel: w575 -> [_ _ _ _ _ _ w746]
          tunnel: [_ _ _ _ _ _ w742] -> w574
          frame #0 {
            n223 = call "Heater_Enable_Chs.vi"() -> ("Inlet Heaters"=w590:T5)  [unwired: 4 in, 5 out]
            n224 = Unbundle By Name(w590) -> ("Connected Items"=w589:string[])
            n225 = for {
              tunnel: w589 -> [w597] mode=indexing
              tunnel: w588 -> [w596]
              tunnel: w587 -> [w595]
              tunnel: [w594] -> w586 mode=indexing
              tunnel: [w593] -> w582 mode=indexing
              n226 = call "Read_value_of_earlier_Ch.vi"("Desired Ch to Read"=w597, "Ch names"=w595, "Present scan array"=w596) -> ("Value"=w594:dbl, "Scan comment"=w593:string)  [unwired: 1 in]
            }
            n227 = Add Array Elements(numeric array=w586) -> (sum=w585:dbl)
            n228 = Greater Than 0?(x=w585) -> (x > 0?=w584:bool)
            n229 = case shown="True" w584 {
              tunnel: [string[] [] ("Sub set") string[] ["EnFlo_Tunnel:Temp:Inlet_Y=0_Z=50", "EnFlo_Tunnel:Temp:Inlet_Y=0_Z=150", "EnFlo_Tunnel:Temp:Inlet_Y=0_Z=250", "EnFlo_Tunnel:Temp:Inlet_Y=0_Z=350", "EnFlo_Tunnel:Temp:Inlet_Y=0_Z=450", "EnFlo_Tunnel:Temp:Inlet_Y=0_Z=550", "EnFlo_Tunnel:Temp:Inlet_Y=0_Z=650", "EnFlo_Tunnel:Temp:Inlet_Y=0_Z=750", "EnFlo_Tunnel:Temp:Inlet_Y=0_Z=850", "EnFlo_Tunnel:Temp:Inlet_Y=0_Z=950", "EnFlo_Tunnel:Temp:Inlet_Y=0_Z=1050", "EnFlo_Tunnel:Temp:Inlet_Y=0_Z=1150", "EnFlo_Tunnel:Temp:Inlet_Y=0_Z=1250", "EnFlo_Tunnel:Temp:Inlet_Y=0_Z=1350", "EnFlo_Tunnel:Temp:Inlet_Y=0_Z=1450"] ("Sub set")] -> w583
              frame False {
              }
              frame True {
              }
            }
          }
          frame #1 {
            w599 = 750.0 ("Y Scale.Offset and Multiplier:Multiplier")
            w598 = 0.0 ("Y Scale.Offset and Multiplier:Offset")
            w601 = 875.0 ("X Scale.Offset and Multiplier:Multiplier")
            w600 = -1750.0 ("X Scale.Offset and Multiplier:Offset")
            n230 = Initialize Array(0.0, 2 ("dimension size"), 4 ("dimension size")) -> (w602:dbl[][])
            n231 = property on="Temperature" class="IntGraph (strict)"("XScale.Multiplier"=w601, "XScale.Offset"=w600, "YScale.Multiplier"=w599, "YScale.Offset"=w598) -> ()  [unwired: 2 in, 2 out]
            n232 = property on="Power" class="IntGraph (strict)"("XScale.Multiplier"=w601, "XScale.Offset"=w600, "YScale.Multiplier"=w599, "YScale.Offset"=w598) -> ()  [unwired: 2 in, 2 out]
          }
          frame #2 {
            n233 = for {
              N: 8 -> [_]
              tunnel: [w618] -> w611 mode=indexing
              tunnel: [w614] -> w608 mode=concatenating
              i -> [w617]
              n234 = Increment(x=w617) -> (x+1=w616:i32)
              n235 = case shown="7" w616 {
                tunnel: [string[] ["EnFlo_Tunnel:Temp:Inlet_Y=-1500_Z=950", "EnFlo_Tunnel:Temp:Inlet_Y=-1000_Z=950", "EnFlo_Tunnel:Temp:Inlet_Y=-1500_Z=1450", "EnFlo_Tunnel:Temp:Inlet_Y=-1000_Z=1450"] ("subarray") string[] ["EnFlo_Tunnel:Temp:Inlet_Y=-1500_Z=50", "EnFlo_Tunnel:Temp:Inlet_Y=-1000_Z=50", "EnFlo_Tunnel:Temp:Inlet_Y=-1500_Z=450", "EnFlo_Tunnel:Temp:Inlet_Y=-1000_Z=450"] ("subarray") string[] ["EnFlo_Tunnel:Temp:Inlet_Y=-500_Z=950", "EnFlo_Tunnel:Temp:Inlet_Y=0_Z=950", "EnFlo_Tunnel:Temp:Inlet_Y=-500_Z=1450", "EnFlo_Tunnel:Temp:Inlet_Y=0_Z=1450"] ("subarray") string[] ["EnFlo_Tunnel:Temp:Inlet_Y=-500_Z=50", "EnFlo_Tunnel:Temp:Inlet_Y=0_Z=50", "EnFlo_Tunnel:Temp:Inlet_Y=-500_Z=450", "EnFlo_Tunnel:Temp:Inlet_Y=0_Z=450"] ("subarray") string[] ["EnFlo_Tunnel:Temp:Inlet_Y=500_Z=950", "EnFlo_Tunnel:Temp:Inlet_Y=0_Z=950", "EnFlo_Tunnel:Temp:Inlet_Y=500_Z=1450", "EnFlo_Tunnel:Temp:Inlet_Y=0_Z=1450"] ("subarray") string[] ["EnFlo_Tunnel:Temp:Inlet_Y=500_Z=50", "EnFlo_Tunnel:Temp:Inlet_Y=0_Z=50", "EnFlo_Tunnel:Temp:Inlet_Y=500_Z=450", "EnFlo_Tunnel:Temp:Inlet_Y=0_Z=450"] ("subarray") string[] ["EnFlo_Tunnel:Temp:Inlet_Y=1500_Z=950", "EnFlo_Tunnel:Temp:Inlet_Y=1000_Z=950", "EnFlo_Tunnel:Temp:Inlet_Y=1500_Z=1450", "EnFlo_Tunnel:Temp:Inlet_Y=1000_Z=1450"] ("subarray") string[] ["EnFlo_Tunnel:Temp:Inlet_Y=1500_Z=50", "EnFlo_Tunnel:Temp:Inlet_Y=1000_Z=50", "EnFlo_Tunnel:Temp:Inlet_Y=1500_Z=450", "EnFlo_Tunnel:Temp:Inlet_Y=1000_Z=450"] ("subarray")] -> w614
                tunnel: [dbl[] [1.0, 1.0, 1.0, 1.0] ("subarray") dbl[] [1.0, 1.0, 1.0, 1.0] ("subarray") dbl[] [1.0, 0.5, 1.0, 0.5] ("subarray") dbl[] [1.0, 0.5, 1.0, 0.5] ("subarray") dbl[] [1.0, 0.5, 1.0, 0.5] ("subarray") dbl[] [1.0, 0.5, 1.0, 0.5] ("subarray") dbl[] [1.0, 1.0, 1.0, 1.0] ("subarray") dbl[] [1.0, 1.0, 1.0, 1.0] ("subarray")] -> w619
                tunnel: ["EnFlo_Tunnel:Inlet_Lamp Y=-1313_Z=1125:Dem_Power(%)" ("Ch Name") "EnFlo_Tunnel:Inlet_Lamp Y=-1313_Z=375:Dem_Power(%)" ("Ch Name") "EnFlo_Tunnel:Inlet_Lamp Y=-438_Z=1125:Dem_Power(%)" ("Ch Name") "EnFlo_Tunnel:Inlet_Lamp Y=-438_Z=375:Dem_Power(%)" ("Ch Name") "EnFlo_Tunnel:Inlet_Lamp Y=438_Z=1125:Dem_Power(%)" ("Ch Name") "EnFlo_Tunnel:Inlet_Lamp Y=438_Z=375:Dem_Power(%)" ("Ch Name") "EnFlo_Tunnel:Inlet_Lamp Y=1313_Z=1125:Dem_Power(%)" ("Ch Name") "EnFlo_Tunnel:Inlet_Lamp Y=1313_Z=375:Dem_Power(%)" ("Ch Name")] -> w615
                tunnel: [1 0 1 0 1 0 1 0] -> w613
                tunnel: [0 0 1 1 2 2 3 3] -> w612
                frame 1, Default {
                }
                frame 2 {
                }
                frame 3 {
                }
                frame 4 {
                }
                frame 5 {
                }
                frame 6 {
                }
                frame 7 {
                }
                frame 8 {
                }
              }
              n236 = Bundle("Ch Name"=w615, "subarray"=w614, "subarray"=w619, w613, w612) -> (w618:T6)  [unwired: 1 in]
            }
            n237 = Build Array (concatenate)(w607, w608) -> (w606:string[])
            n238 = call "Analyse_string_array.vi"("String array"=w606) -> ("Unique strings"=w609:string[])  [unwired: 1 in, 1 out]
          }
          frame #3 {
            # "Averaging time seconds"
            n239 = Subtract(x=w665, y=w664) -> (x-y=w669:dbl)
            n240 = call "Get_ADAM_averages_server.vi"("No of averages"=1, "End time"=w665, "Start time"=w669, "Clients time"=w665, "ADAM Ch Names"=w663) -> ("DBL values"=w667:dbl[][])  [unwired: 1 in, 4 out]
            n241 = Index Array(array=w667, index (row)=0) -> (element=w662:dbl[])  [unwired: 1 in]
            n242 = Array Subset(array=w662, index=1) -> (w660:dbl[])  [unwired: 1 in]
          }
          frame #4 {
            n243 = case shown="True" w674 {
              tunnel: w673 -> [_ w679]
              tunnel: w672 -> [_ w678]
              tunnel: w671 -> [_ w677]
              tunnel: [dbl[] [] w676] -> w670
              frame False {
              }
              frame True {
                n244 = for {
                  tunnel: w679 -> [w683]
                  tunnel: w678 -> [w682] mode=indexing
                  tunnel: w677 -> [w681]
                  tunnel: [w680] -> w676 mode=indexing
                  n245 = Search 1D Array(1D array=w683, element=w682) -> (index of element=w684:i32)  [unwired: 1 in]
                  n246 = Index Array(array=w681, index=w684) -> (element=w680:dbl)
                }
              }
            }
          }
          frame #5 {
            n247 = for {
              tunnel: w700 -> [w715] mode=indexing
              tunnel: w699 -> [w714]
              tunnel: w698 -> [w712]
              tunnel: [w703] -> w691 mode=indexing
              shift-right: [w706] -> w696
              shift-left: w697 -> [w707]
              tunnel: w686 -> [w702]
              tunnel: w685 -> [w701]
              n248 = Unbundle(w715) -> ("subarray"=w713:string[], "subarray"=w711:dbl[], w705:i32, w704:i32)  [unwired: 1 out]
              n249 = for {
                tunnel: w714 -> [w725]
                tunnel: w713 -> [w717] mode=indexing
                tunnel: w712 -> [w724]
                tunnel: w711 -> [w722] mode=indexing
                tunnel: [w721] -> w710 mode=indexing
                tunnel: w702 -> [w720]
                tunnel: w701 -> [w716]
                n250 = Search 1D Array(1D array=w725, element=w717) -> (index of element=w723:i32)  [unwired: 1 in]
                n251 = Index Array(array=w724, index=w723) -> (element=w718:dbl)
                n252 = case shown="True" w720 {
                  tunnel: [w726 w727] -> w719
                  tunnel: w718 -> [w726 w729]
                  tunnel: w717 -> [_ w741]
                  tunnel: w716 -> [_ w730]
                  frame False {
                  }
                  frame True {
                    n253 = Reverse String(1:w741) -> (0:w740:string)
                    n254 = Match Pattern(string=w740, regular expression="=") -> (before substring=w738:string)  [unwired: 1 in, 3 out]
                    n255 = Reverse String(1:w738) -> (0:w737:string)
                    n256 = Fract/Exp String To Number(string=w737) -> (number=w736:dbl)  [unwired: 3 in, 1 out]
                    n257 = Subtract(x=w736, y=50.0) -> (x-y=w734:dbl)
                    n258 = Divide(x=w734, y=100.0) -> (x/y=w732:dbl)
                    n259 = To Long Integer(number=w732) -> (32bit integer=w731:i32)
                    n260 = Index Array(array=w730, index=w731) -> (element=w728:dbl)
                    n261 = Subtract(x=w729, y=w728) -> (x-y=w727:dbl)
                  }
                }
                n262 = Multiply(x=w719, y=w722) -> (x*y=w721:dbl)
              }
              n263 = Add Array Elements(numeric array=w711) -> (sum=w708:dbl)
              n264 = Add Array Elements(numeric array=w710) -> (sum=w709:dbl)
              n265 = Divide(x=w709, y=w708) -> (x/y=w703:dbl)
              n266 = Replace Array Subset(array=w707, new element=w703, index (row)=w705, index (col)=w704) -> (w706:dbl[][])
            }
            "Temperature" <- w696
            n267 = Array Max & Min(array=w691) -> (max value=w689:dbl, min value=w688:dbl)  [unwired: 2 out]
            n268 = Subtract(x=w689, y=w688) -> (x-y=→"Max Delta T":dbl)
            n269 = Bundle(w689, u32 16721152) -> (w694:cluster{dbl, u32})  [unwired: 1 out]
            n270 = Bundle(w688, u32 3743) -> (w695:cluster{dbl, u32})  [unwired: 1 out]
            n271 = Build Array(w694, w695) -> (w690:cluster{dbl, u32}[])
            n272 = property on="Temperature" class="IntGraph (strict)"("ZScale.MarkerVals[]"=w690) -> ()  [unwired: 2 in, 2 out]
          }
          frame #6 {
            n273 = Array Max & Min(array=w763) -> (max value=w764:dbl)  [unwired: 3 out]
            n274 = for {
              tunnel: w774 -> [w802] mode=indexing
              tunnel: w773 -> [w801]
              tunnel: w772 -> [w800]
              tunnel: w764 -> [w788]
              tunnel: "Kp Lamps" -> [w795]
              tunnel: [w790] -> w768 mode=indexing
              tunnel: [w789] -> w760 mode=indexing
              tunnel: w763 -> [w787] mode=indexing
              tunnel: [w786] -> w762 mode=indexing
              tunnel: [w785] -> w756 mode=indexing
              tunnel: [w784] -> w755 mode=indexing
              tunnel: [w783] -> w744 mode=indexing
              n275 = Unbundle(w802) -> ("Ch Name"=w789:string, w785:i32, w784:i32)  [unwired: 2 out]
              n276 = call "Read_value_of_earlier_Ch.vi"("Desired Ch to Read"=w789, "Ch names"=w800, "Present scan array"=w801) -> ("Value"=w786:dbl, "Scan comment"=w783:string)  [unwired: 1 in]
              n277 = Subtract(x=w788, y=w787) -> (x-y=w794:dbl)
              n278 = Multiply(x=w795, y=w794) -> (x*y=w796:dbl)
              n279 = In Range and Coerce(upper limit=8.0, x=w796, lower limit=-8.0) -> (coerced(x)=w799:dbl)  [unwired: 1 out]
              n280 = Add(x=w786, y=w799) -> (x+y=w791:dbl)
              n281 = Not A Number/Path/Refnum?(number/path/refnum=w791) -> (NaN/Path/Refnum?=w792:bool)
              n282 = Select(t=0.0, s=w792, f=w791) -> (s? t:f=w790:dbl)
            }
            n283 = Array Max & Min(array=w768) -> (min value=w767:dbl)  [unwired: 3 out]
            n284 = Subtract(x=w768, y=w767) -> (x-y=w766:dbl[])
            n285 = In Range and Coerce(upper limit=100.0, x=w766, lower limit=0.0) -> (coerced(x)=w761:dbl[])  [unwired: 1 out]
            n286 = for {
              tunnel: w762 -> [w782] mode=indexing
              tunnel: w761 -> [w775] mode=indexing
              tunnel: [w781] -> w759 mode=indexing if=w780
              tunnel: w760 -> [w781] mode=indexing
              tunnel: [w775] -> w758 mode=indexing if=w780
              shift-right: [w778] -> w748
              shift-left: w757 -> [w779]
              tunnel: w756 -> [w777] mode=indexing
              tunnel: w755 -> [w776] mode=indexing
              n287 = Replace Array Subset(array=w779, new element=w775, index (row)=w777, index (col)=w776) -> (w778:dbl[][])
              n288 = Not Equal?(x=w775, y=w782) -> (x != y?=w780:bool)
            }
            "Power" <- w748
            n289 = Array Max & Min(array=w748) -> (max value=w750:dbl, min value=w749:dbl)  [unwired: 2 out]
            n290 = Bundle(w750, u32 16721152) -> (w753:cluster{dbl, u32})  [unwired: 1 out]
            n291 = Bundle(w749, u32 3743) -> (w754:cluster{dbl, u32})  [unwired: 1 out]
            n292 = Build Array(w753, w754) -> (w747:cluster{dbl, u32}[])
            n293 = property on="Power" class="IntGraph (strict)"("ZScale.MarkerVals[]"=w747) -> ()  [unwired: 2 in, 2 out]
            n294 = call "ASYNC_Adam_server.vi"("Values"=w758, "Channel Names"=w759) -> ("Scan Comments"=w743:string[])  [unwired: 1 in, 2 out]
            n295 = Concatenate Strings(w746, w745, w744, w743) -> (w742:string)
          }
        }
      }
      frame "Check EnFlo tweak factor?" {
        n296 = global read "ADAM_Global.vi" "Client State Array"() -> (w806:T7[])
        n297 = for {
          tunnel: w806 -> [w817] mode=indexing
          tunnel: [w810] -> w804
          stop <- w811 stop-if-true
          n298 = Unbundle By Name(w817) -> ("Client Name"=w813:string, "Traverse level State"=w816:T4)
          n299 = Equal?(x=w816, y=Traverse_Level_State."Running" ("Traverse level State")) -> (x = y?=w810:bool)
          n300 = Equal?(x="EnFlo_Tunnel" ("y"), y=w813) -> (x = y?=w812:bool)
          n301 = And(x=w812, y=w810) -> (x .and. y?=w811:bool)
        }
        n302 = case shown="True" w804 {
          tunnel: ["Lab Temp Control" "Are Inlet Screens Blocked?"] -> w805
          frame False {
          }
          frame True {
          }
        }
      }
      frame "Are Inlet Screens Blocked?" {
        n303 = stacked-sequence {
          seq-local: [w821 _] -> [_ w836]
          seq-local: [w824 _] -> [_ w835]
          frame #0 {
            n304 = Build Array("Status:of:EnFlo_Tunnel", "EnFlo_Tunnel:Inlet:K_Factor") -> (w826:string[])
            n305 = call "Get_Channel_averages.vi"("Desired Ch Names"=w826, "Averaging time (mins)"=60.0) -> ("number"=w832:dbl[])  [unwired: 1 in, 2 out]
            n306 = Index Array(array=w832, index=1) -> (element=w821:dbl)
            n307 = Index Array(array=w832, index=0) -> (element=w831:dbl)
            n308 = Greater?(x=w821, y="Max K Factor") -> (0:w823:bool)
            n309 = Equal?(x=w831, y=2.0) -> (x = y?=w829:bool)
            n310 = Compound Arithmetic op=AND(w823, w829) -> (w824:bool)
          }
          frame #1 {
            n311 = case shown="True" w835 {
              tunnel: w836 -> [_ w840]
              frame False {
              }
              frame True {
                n312 = Format Into String(format string="The Inlet K factor for the EnFlo Tunnel is now %.2f. This may indicate that the screens need cleaning." ("Format String"), w840) -> (resulting string=w838:string)  [unwired: 2 in, 1 out]
                n313 = call "Server_Emails.vi"("Client Name Contains"="EnFlo_Tunnel", "Message"=w838, "Subject"="EnFlo Tunnel Screens" ("Message")) -> ()  [unwired: 2 in, 3 out]
              }
            }
          }
        }
      }
      frame "Lab Temp Control" {
        n314 = call "EnFlo_Lab_Temp_Control.vi"("Current Time"=w843) -> ()
      }
      frame "Is Dew point meter Alive?" {
        n315 = Build Array (concatenate)(w864, string[] ["EnFlo_Tunnel:Chiller_Pump:Running", "EnFlo_Tunnel:Floor_Cooling:Enable"] ("appended array")) -> (w863:string[])
        n316 = call "Read_Earlier_Channels.vi"("Present scan array"=w866, "Ch names"=w865, "Desired Channels"=w863) -> ("Scan comments"=w847:string, "Index 0"=w862:dbl, "Index 1"=w861:dbl, "Index 2"=w852:dbl)  [unwired: 2 out]
        n317 = Not A Number/Path/Refnum?(number/path/refnum=w862) -> (NaN/Path/Refnum?=w858:bool)
        n318 = Greater?(x=w852, y=0.5) -> (0:w851:bool)
        n319 = Greater?(x=w861, y=0.5) -> (0:w860:bool)
        n320 = while {
          tunnel: [w871] -> w856
          tunnel: [w872] -> w857
          shift-left: _ -> [w872]
          tunnel: w858 -> [w873]
          shift-left: _ -> [w871]
          shift-right: [w873] -> _
          stop <- FALSE continue-if-true
        }
        n321 = Compound Arithmetic op=AND(invert w858, w860, w851) -> (w859:bool)
        n322 = Compound Arithmetic op=AND(w856, invert w857, w858) -> (w867:bool)
        n323 = case shown="True" w867 {
          frame False {
          }
          frame True {
            w874 = TRUE  # Contact All clients?
            n324 = call "Server_Emails.vi"("Message"="The humidity meter is not communicating with the server.\nIt can be reset by switching the toggle switch off and then on again after about 15 seconds." ("Bundle Element"), "Contact All clients?"=w874, "Subject"="Humidity Meter Offline" ("Error Type")) -> ()  [unwired: 2 in, 3 out]
          }
        }
        n325 = Select(t="Condensation Alert 1", s=w859, f="More checks") -> (s? t:f=w869:string)
        n326 = Concatenate Strings(w848, w847) -> (w846:string)
      }
      frame "Condensation Alert 1" {
        w884 = "EnFlo Lab:Hygrometry:Dew Point temp_PN"
        w886 = "EnFlo_Tunnel:Chilled Water:Dem Temp"
        n327 = Build Array(w884, w886) -> (w891:string[])
        n328 = while {
          tunnel: [w899] -> w887
          tunnel: [w900] -> w890
          shift-left: _ -> [w900]
          shift-right: [w896] -> w889
          tunnel: w891 -> [w905]
          tunnel: w892 -> [w906]
          tunnel: w893 -> [w907]
          tunnel: [w897] -> w885
          tunnel: [w896] -> w883
          tunnel: [w895] -> w877 mode=indexing
          stop <- FALSE continue-if-true
          n329 = call "Read_Earlier_Channels.vi"("Present scan array"=w907, "Ch names"=w906, "Desired Channels"=w905) -> ("Scan comments"=w895:string, "Index 0"=w899:dbl, "Index 1"=w897:dbl)  [unwired: 3 out]
          n330 = Select(t=1.5, s=w900, f=0.5) -> (s? t:f=w901:dbl)
          n331 = Add(x=w899, y=w901) -> (x+y=w904:dbl)
          n332 = Greater?(x=w904, y=w897) -> (0:w896:bool)
        }
        n333 = Compound Arithmetic op=AND(invert w890, w889) -> (w888:bool)
        n334 = case shown="True" w888 {
          tunnel: w887 -> [_ w911]
          tunnel: w886 -> [_ w910]
          tunnel: w885 -> [_ w909]
          tunnel: w884 -> [_ w908]
          frame False {
          }
          frame True {
            n335 = Format Into String(format string="The %s is %.1f deg C  and the %s is %.1f. \n\nCondensation on the tunnel floor or in the heat exchanger could be occuring." ("Format String"), w908, w911, w910, w909) -> (resulting string=w913:string)  [unwired: 2 in, 1 out]
            n336 = call "Server_Emails.vi"("Client Name Contains"="EnFlo_Tunnel", "Message"=w913, "Subject"="Condensation Alert1" ("Error Type")) -> ()  [unwired: 2 in, 3 out]
          }
        }
        n337 = Select(t="Condensation Alert 2", s=w883, f="More checks") -> (s? t:f=w880:string)
        n338 = Concatenate Strings(w879, w877) -> (w878:string)
      }
      frame "Condensation Alert 2" {
        w920 = "EnFlo Lab:Hygrometry:Dew Point temp_PN"
        w922 = "EnFlo_Tunnel:Chilled Water:Dem Temp"
        n339 = Build Array(w920, w922) -> (w927:string[])
        n340 = while {
          tunnel: [w935] -> w923
          tunnel: [w936] -> w926
          shift-left: _ -> [w936]
          shift-right: [w932] -> w925
          tunnel: w927 -> [w941]
          tunnel: w928 -> [w942]
          tunnel: w929 -> [w943]
          tunnel: [w933] -> w921
          tunnel: [w931] -> w916 mode=indexing
          stop <- FALSE continue-if-true
          n341 = call "Read_Earlier_Channels.vi"("Present scan array"=w943, "Ch names"=w942, "Desired Channels"=w941) -> ("Scan comments"=w931:string, "Index 0"=w935:dbl, "Index 1"=w933:dbl)  [unwired: 3 out]
          n342 = Select(t=0.5, s=w936, f=-0.5) -> (s? t:f=w937:dbl)
          n343 = Add(x=w935, y=w937) -> (x+y=w940:dbl)
          n344 = Greater?(x=w940, y=w933) -> (0:w932:bool)
        }
        n345 = Compound Arithmetic op=AND(invert w926, w925) -> (w924:bool)
        n346 = case shown="True" w924 {
          tunnel: w923 -> [_ w947]
          tunnel: w922 -> [_ w946]
          tunnel: w921 -> [_ w945]
          tunnel: w920 -> [_ w944]
          frame False {
          }
          frame True {
            n347 = Format Into String(format string="The %s is %.1f deg C  and the %s is %.1f. \n\nCondensation on the tunnel floor or in the heat exchanger could well be occuring." ("Format String"), w944, w947, w946, w945) -> (resulting string=w949:string)  [unwired: 2 in, 1 out]
            n348 = call "Server_Emails.vi"("Client Name Contains"="EnFlo_Tunnel", "Message"=w949, "Subject"="Condensation Alert2" ("Error Type")) -> ()  [unwired: 2 in, 3 out]
          }
        }
        n349 = Concatenate Strings(w918, w916) -> (w917:string)
      }
      frame "More checks" {
        n350 = Build Array("Fast FID:Valco Valve:Position", "Status:of:EnFlo_Tunnel") -> (w965:string[])
        n351 = call "Read_Earlier_Channels.vi"("Present scan array"=w969, "Ch names"=w968, "Desired Channels"=w965) -> ("Scan comments"=w954:string, "Index 0"=w958:dbl)  [unwired: 4 out]
        n352 = Equal?(x=4.0, y=w958) -> (x = y?=w962:bool)
        n353 = Equal?(x=1.0, y=w958) -> (x = y?=w961:bool)
        n354 = Not A Number/Path/Refnum?(number/path/refnum=w958) -> (NaN/Path/Refnum?=w963:bool)
        n355 = Compound Arithmetic op=OR(w961, w962, w963) -> (w960:bool)
        n356 = Select(t="End", s=w960, f="Set FFID Valve to Measure") -> (s? t:f=w966:string)
        n357 = Concatenate Strings(w953, w954) -> (w952:string)
      }
      frame "Set FFID Valve to Measure" {
        w992 = FALSE  # All Active Channels
        n358 = Build Array("Fast FID:Valco Valve:Position") -> (w990:string[])
        n359 = call "Channel_Names_and_indicies.vi"("All Active Channels"=w992, "Desired Ch Names"=w990) -> ("Indicies"=w991:i32[])  [unwired: 1 out]
        n360 = Subtract(x=w993, y=700.0) -> (x-y=w988:dbl)
        n361 = call "Specified_Channels_server.vi"("End time"=w993, "Start time"=w988, "Clients time"=w993, "Requested channels"=w991) -> ("Output array"=w985:dbl[][], "Messages"=w972:string)  [unwired: 1 in, 3 out]
        n362 = Index Array(array=w985, index (row)=0 ("Index")) -> (element=w981:dbl[])  [unwired: 1 in]
        n363 = Not A Number/Path/Refnum?(number/path/refnum=w981) -> (NaN/Path/Refnum?=w980:bool[])
        n364 = Or Array Elements(Boolean array=w980) -> (logical OR=w978:bool)
        n365 = Array Max & Min(array=w981) -> (max value=w983:dbl, min value=w984:dbl)  [unwired: 2 out]
        n366 = Subtract(x=w983, y=w984) -> (x-y=w982:dbl)
        n367 = Equal To 0?(x=w982) -> (x = 0?=w979:bool)
        n368 = Compound Arithmetic op=AND(w979, invert w978) -> (w977:bool)
        n369 = case shown="True" w977 {
          tunnel: w976 -> [_ w1001]
          tunnel: w975 -> [_ w1000]
          frame False {
          }
          frame True {
            n370 = Build Array("FFID:System:Enable") -> (w998:string[])
            n371 = call "Read_Earlier_Channels.vi"("Present scan array"=w1000, "Ch names"=w1001, "Desired Channels"=w998) -> ("Index 0"=w997:dbl)  [unwired: 5 out]
            n372 = Greater?(x=w997, y=0.5) -> (0:w995:bool)
            n373 = case shown="True" w995 {
              frame False {
                n374 = Build Array(0.0) -> (w1002:dbl[])
                n375 = Build Array("GMU:Gas:Enable") -> (w1003:string[])
                n376 = call "ASYNC_Adam_server.vi"("Values"=w1002, "Channel Names"=w1003) -> ()  [unwired: 1 in, 3 out]
              }
              frame True {
                w1006 = T8 4 items=["", "Zero Air", "Calib 1", "Calib 2", "Measure"] ("Requested Position")
                n377 = call "Fast_FID_Valve_Control.vi"("Requested Position"=w1006) -> ()  [unwired: 7 out]
              }
            }
          }
        }
        n378 = Concatenate Strings(w973, w972) -> (w971:string)
      }
      frame "End" {
        n379 = stacked-sequence {
          seq-local: [w1028 _ _] -> [_ w1049 _]
          seq-local: [w1022 _ _] -> [_ w1046 _]
          tunnel: w1016 -> [w1033 _ _]
          tunnel: w1015 -> [w1025 w1048 w1067]
          tunnel: w1014 -> [w1026 w1047 w1068]
          tunnel: w1013 -> [_ _ w1063]
          tunnel: [_ _ w1060] -> w1011
          tunnel: [_ _ w1059] -> w1010
          tunnel: [w1021 _ _] -> w1009
          frame #0 {
            n380 = call <vilib>:"LV70TimeStampToDateRec.vi"("time stamp"=w1033) -> ("date time rec"=w1034:T9)
            n381 = Unbundle By Name(w1034) -> ("hour"=w1032:i32, "day of week"=w1031:i32, "year"=w1020:i32)
            n382 = Greater?(x=w1020, y=2017) -> (0:w1018:bool)
            n383 = while {
              tunnel: w1032 -> [w1045]
              tunnel: w1031 -> [w1043]
              shift-right: [w1038] -> w1029
              shift-left: _ -> [w1037]
              tunnel: [w1037] -> w1030
              tunnel: w1018 -> [w1035]
              stop <- FALSE continue-if-true
              n384 = Equal?(x=w1045, y=10) -> (x = y?=w1039:bool)
              n385 = In Range and Coerce(upper limit=7, x=w1043, lower limit=1) -> (In Range?=w1040:bool)  [unwired: 1 out]
              n386 = Compound Arithmetic op=AND(w1039, w1040, w1035) -> (w1038:bool)
            }
            n387 = call "Read_value_of_earlier_Ch.vi"("Desired Ch to Read"="Uni:Chilled Water:Temp", "Ch names"=w1025, "Present scan array"=w1026) -> ("Value"=w1022:dbl, "Scan comment"=w1021:string)  [unwired: 1 in]
            n388 = Greater?(x=w1022, y=15.0) -> (0:w1023:bool)
            n389 = Compound Arithmetic op=AND(w1023, invert w1030, w1029) -> (w1028:bool)
          }
          frame #1 {
            n390 = case shown="True" w1049 {
              tunnel: w1048 -> [_ _]
              tunnel: w1047 -> [_ _]
              tunnel: w1046 -> [_ w1057]
              frame False {
              }
              frame True {
                n391 = Select(t=string[] [], s="Disable Sending email to estates regarding Chilled water Temp", f=string[] ["efmenquiries@surrey.ac.uk"] ("Extra People to Email")) -> (s? t:f=w1050:string[])
                n392 = Format Into String(format string="Dear Estates\n\nThe monitoring system in the EnFlo Lab (01AB01) is currently indicating that the Chilled water in the AB Building is at %d deg C.\n\nPlease could you arrange for somebody to come and investigate this please.\n\nThanks very much\n\nPaul Hayden x9545  or Mobile  07961 608409", w1057) -> (resulting string=w1056:string)  [unwired: 2 in, 1 out]
                n393 = call "Server_Emails.vi"("Message"=w1056, "Contact All clients?"=TRUE, "Subject"="Chilled water in AB Building above 15 deg C" ("Error Type"), "Extra People to Email"=w1050) -> ()  [unwired: 1 in, 3 out]
              }
            }
          }
          frame #2 {
            w1061 = "Aero_Tunnel:Seeder:Enable" ("Desired Ch to Read")
            n394 = call "Read_value_of_earlier_Ch.vi"("Desired Ch to Read"=w1061, "Ch names"=w1067, "Present scan array"=w1068) -> ("Value"=w1066:dbl)  [unwired: 1 in, 1 out]
            n395 = Greater?(x=w1066, y=0.5) -> (0:w1064:bool)
            n396 = case shown="False" w1064 {
              tunnel: w1061 -> [_ w1083]
              tunnel: w1063 -> [_ w1082]
              tunnel: [FALSE w1078] -> w1062
              tunnel: ["" w1077] -> w1059
              frame False {
              }
              frame True {
                w1090 = FALSE  # All Active Channels
                n397 = Build Array(w1083) -> (w1088:string[])
                n398 = call "Channel_Names_and_indicies.vi"("All Active Channels"=w1090, "Desired Ch Names"=w1088) -> ("Indicies"=w1089:i32[])  [unwired: 1 out]
                n399 = Subtract(x=w1082, y=30.0) -> (x-y=w1086:dbl)
                n400 = call "Specified_Channels_server.vi"("End time"=w1082, "Start time"=w1086, "Clients time"=w1082, "Requested channels"=w1089) -> ("Output array"=w1084:dbl[][], "Messages"=w1077:string)  [unwired: 1 in, 3 out]
                n401 = Index Array(array=w1084, index (row)=0 ("Index")) -> (element=w1080:dbl[])  [unwired: 1 in]
                n402 = Greater?(x=w1080, y=0.5) -> (0:w1079:bool[])
                n403 = And Array Elements(Boolean array=w1079) -> (logical AND=w1078:bool)
              }
            }
            n404 = case shown="False" w1062 {
              tunnel: w1061 -> [_ w1074]
              tunnel: ["" w1070] -> w1060
              frame False {
              }
              frame True {
                n405 = Build Array(w1074) -> (w1073:string[])
                n406 = call "ASYNC_Adam_server.vi"("Values"=dbl[] [0.0], "Channel Names"=w1073) -> ("Scan Comments"=w1071:string[])  [unwired: 1 in, 2 out]
                n407 = Concatenate Strings(w1071) -> (w1070:string)
              }
            }
          }
        }
        n408 = Concatenate Strings(w1008, w1009, w1011, w1010) -> (w1007:string)
      }
      frame "No Match", Default {
        n409 = Current VI's Path() -> (path=w1095:path)
        n410 = Format Into String(format string="The Case\"%s\" was not Matched\nin VI named\n'%s\"" ("Format String"), w1094, w1095) -> (resulting string=w1098:string)  [unwired: 2 in, 1 out]
        n411 = One Button Dialog(message=w1098, button name ("OK")="STOP") -> (true=w1096:bool)
        n412 = Stop(stop? (T)=w1096) -> ()
      }
    }
  }
  "Scan Comments" <- w1
